vi "Autonomous Independent.vi"() -> ()   [LabVIEW 2016]
doc: "This VI is called when autonomous begins, and will automatically be terminated when autonomous ends. You can carry out timed or sensor driven robot movement independently without needing to return to the caller."
uses:
  AutoStates.ctl
  <vilib>/Platform/TimedLoop/XDataNode/timing_clust.ctl
  <vilib>/Platform/TimedLoop/XDataNode/nitl_modes.ctl
  <vilib>/Platform/TimedLoop/XDataNode/wakeup.ctl
  GearPositions.ctl
  Drive Commands.ctl
  Gear Command.ctl
  <vilib>/Rock Robotics/Network Tables/NT Read Number.vi
  <vilib>/Rock Robotics/Network Tables/NT Read Boolean.vi
  <vilib>/addons/control/pid/pid.llb/PID (DBL).vi
  <vilib>/platform/TimedLoop/XDataNode/XDataNode.xnode
  <vilib>/addons/control/pid/NI_PID_pid.lvlib
  <vilib>/Platform/TimedLoop/XDataNode/XDNodeRunTimeDep.lvlib
panel:
  in  "Orientation Limit":dbl=30.0
  out "Waveform Chart":cluster{i16, i16, i16}(graph)={1, 0, 0}
  in  "Drive Path Control":T1={"X"=[0.0, 26.0], "Y"=[0.0, 91.0], "Absolute Theta initial"=1.570796, "Absolute Theta final"=0.5016, "Amount of Time (s) 2"=3.0} {"Amount of Time (s) 2" format="%#_13g"}
  out "Arc Lenth Chart 2":cluster{dbl, "setpoint":dbl}(graph)={164.08658624999998, "setpoint"=169.64378866586094}
  out "Angle Chart (rad) 2":cluster{"Yaw Wind":dbl, "setpoint":dbl}(graph)={"Yaw Wind"=3.171890843977217, "setpoint"=3.2044361193738906}
  in  "Speed Range 2":cluster{"output high":dbl, "output low":dbl}={"output high"=1.0, "output low"=-1.0} {"output low" format="%.2f"; "output high" format="%.2f"}
  in  "PID Speed gains 2":T2={"proportional gain (Kc)"=0.1, "integral time (Ti, min)"=0.0, "derivative time (Td, min)"=0.0} {"derivative time (Td, min)" format="%.3f"; "integral time (Ti, min)" format="%.3f"; "proportional gain (Kc)" format="%.3f"}
  in  "Steer Range 2":cluster{"output high":dbl, "output low":dbl}={"output high"=1.0, "output low"=-1.0} {"output low" format="%.2f"; "output high" format="%.2f"}
  in  "Steer Gains":T2={"proportional gain (Kc)"=1.8, "integral time (Ti, min)"=0.0, "derivative time (Td, min)"=0.0} {"derivative time (Td, min)" format="%.3f"; "integral time (Ti, min)" format="%.3f"; "proportional gain (Kc)" format="%.3f"}
  in  "Eval Period (sec)":dbl(knob)=1.001252153636024 scale=0.0..1.5
  in  "PID Segments (1-500) 2":dbl=60.0
  out "Verify Graph 2":cluster{"X":dbl, "Y":dbl}[](graph)=[{"X"=0.0, "Y"=0.0}, {"X"=0.000288074563179022, "Y"=0.24281266883652286}, {"X"=0.0011475053216401378, "Y"=0.4902662165487718}, {"X"=0.0025713386426217373, "Y"=0.7423268407122737}, {"X"=0.004552620893362211, "Y"=0.9989607389025562}, {"X"=0.007084398441099949, "Y"=1.260134108695146}, {"X"=0.010159717653073339, "Y"=1.5258131476655705}, {"X"=0.013771624896520774, "Y"=1.795964053389357}, {"X"=0.017913166538680646, "Y"=2.0705530234420326}, {"X"=0.022577388946791337, "Y"=2.3495462553991238}, {"X"=0.027757338488091247, "Y"=2.632909946836159}, {"X"=0.03344606152981875, "Y"=2.9206102953286637}, {"X"=0.03963660443921224, "Y"=3.2126134984521664}, {"X"=0.046322013583510145, "Y"=3.5088857537821943}, {"X"=0.053495335329950794, "Y"=3.809393258894274}, {"X"=0.06114961604577262, "Y"=4.1141022113639325}, {"X"=0.06927790209821401, "Y"=4.422978808766698}, {"X"=0.07787323985451333, "Y"=4.735989248678097}, {"X"=0.08692867568190896, "Y"=5.053099728673654}, {"X"=0.09643725594763934, "Y"=5.374276446328901}, {"X"=0.10639202701894285, "Y"=5.699485599219363}, {"X"=0.1167860352630578, "Y"=6.028693384920565}, {"X"=0.1276123270472227, "Y"=6.36186600100804}, {"X"=0.13886394873867589, "Y"=6.698969645057309}, {"X"=0.15053394670465567, "Y"=7.0399705146439}, {"X"=0.1626153673124006, "Y"=7.384834807343345}, {"X"=0.17510125692914894, "Y"=7.733528720731165}, {"X"=0.18798466192213917, "Y"=8.086018452382891}, {"X"=0.20125862865860958, "Y"=8.442270199874049}, {"X"=0.21491620350579863, "Y"=8.802250160780169}, {"X"=0.2289504328309447, "Y"=9.16592453267677}, {"X"=0.24335436300128616, "Y"=9.533259513139388}, {"X"=0.2581210403840614, "Y"=9.904221299743547}, {"X"=0.27324351134650887, "Y"=10.278776090064776}, {"X"=0.2887148222558669, "Y"=10.656890081678597}, {"X"=0.3045280194793739, "Y"=11.038529472160542}, {"X"=0.32067614938426814, "Y"=11.423660459086133}, {"X"=0.33715225833778817, "Y"=11.812249240030901}, {"X"=0.3539493927071724, "Y"=12.204262012570375}, {"X"=0.37106059885965914, "Y"=12.599664974280081}, {"X"=0.38847892316248683, "Y"=12.998424322735545}, {"X"=0.4061974119828937, "Y"=13.400506255512294}, {"X"=0.4242091116881182, "Y"=13.805876970185853}, {"X"=0.44250706864539896, "Y"=14.214502664331752}, {"X"=0.4610843292219742, "Y"=14.626349535525518}, {"X"=0.4799339397850822, "Y"=15.04138378134268}, {"X"=0.49904894670196154, "Y"=15.45957159935876}, {"X"=0.5184223963398505, "Y"=15.88087918714929}, {"X"=0.5380473350659873, "Y"=16.305272742289795}, {"X"=0.5579168092476108, "Y"=16.732718462355802}, {"X"=0.5780238652519589, "Y"=17.16318254492284}, {"X"=0.5983615494462704, "Y"=17.596631187566434}, {"X"=0.6189229081977833, "Y"=18.03303058786211}, {"X"=0.6397009878737363, "Y"=18.4723469433854}, {"X"=0.6606888348413678, "Y"=18.91454645171183}, {"X"=0.6818794954679157, "Y"=19.35959531041692}, {"X"=0.7032660161206189, "Y"=19.807459717076206}, {"X"=0.7248414431667157, "Y"=20.258105869265208}, {"X"=0.7465988229734446, "Y"=20.711499964559465}, {"X"=0.7685312019080436, "Y"=21.16760820053449}, {"X"=0.7906316263377513, "Y"=21.62639677476582}, {"X"=0.812893142629806, "Y"=22.087831884828976}, {"X"=0.8353087971514465, "Y"=22.551879728299486}, {"X"=0.8578716362699106, "Y"=23.018506502752878}, {"X"=0.8805747063524371, "Y"=23.487678405764683}, {"X"=0.9034110537662644, "Y"=23.959361634910426}, {"X"=0.9263737248786306, "Y"=24.43352238776563}, {"X"=0.9494557660567741, "Y"=24.91012686190583}, {"X"=0.9726502236679336, "Y"=25.389141254906548}, {"X"=0.9959501440793475, "Y"=25.870531764343305}, {"X"=1.0193485736582537, "Y"=26.35426458779164}, {"X"=1.0428385587718907, "Y"=26.840305922827067}, {"X"=1.0664131457874975, "Y"=27.32862196702513}, {"X"=1.0900653810723118, "Y"=27.819178917961345}, {"X"=1.1137883109935727, "Y"=28.31194297321124}, {"X"=1.137574981918518, "Y"=28.806880330350346}, {"X"=1.161418440214386, "Y"=29.30395718695419}, {"X"=1.1853117322484152, "Y"=29.803139740598297}, {"X"=1.2092479043878446, "Y"=30.30439418885819}, {"X"=1.233220002999912, "Y"=30.807686729309403}, {"X"=1.2572210744518557, "Y"=31.312983559527456}, {"X"=1.2812441651109145, "Y"=31.820250877087886}, {"X"=1.3052823213443268, "Y"=32.329454879566214}, {"X"=1.3293285895193305, "Y"=32.84056176453797}, {"X"=1.3533760160031636, "Y"=33.35353772957866}, {"X"=1.3774176471630661, "Y"=33.86834897226385}, {"X"=1.4014465293662752, "Y"=34.38496169016904}, {"X"=1.4254557089800295, "Y"=34.90334208086977}, {"X"=1.4494382323715675, "Y"=35.42345634194157}, {"X"=1.4733871459081276, "Y"=35.94527067095994}, {"X"=1.497295495956948, "Y"=36.46875126550043}, {"X"=1.5211563288852672, "Y"=36.993864323138574}, {"X"=1.5449626910603236, "Y"=37.52057604144988}, {"X"=1.5687076288493556, "Y"=38.048852618009896}, {"X"=1.592384188619601, "Y"=38.578660250394115}, {"X"=1.6159854167382997, "Y"=39.1099651361781}, {"X"=1.6395043595726884, "Y"=39.64273347293735}, {"X"=1.6629340634900065, "Y"=40.176931458247424}, {"X"=1.6862675748574918, "Y"=40.712525289683825}, {"X"=1.7094979400423835, "Y"=41.249481164822086}, {"X"=1.7326182054119197, "Y"=41.78776528123773}, {"X"=1.7556214173333384, "Y"=42.3273438365063}, {"X"=1.778500622173878, "Y"=42.868183028203305}, {"X"=1.8012488663007775, "Y"=43.41024905390428}, {"X"=1.8238591960812744, "Y"=43.953508111184746}, {"X"=1.8463246578826074, "Y"=44.49792639762024}, {"X"=1.8686382980720155, "Y"=45.04347011078629}, {"X"=1.8907931630167365, "Y"=45.590105448258406}, {"X"=1.9127822990840087, "Y"=46.13779860761214}, {"X"=1.9345987526410706, "Y"=46.68651578642299}, {"X"=1.9562355700551612, "Y"=47.23622318226651}, {"X"=1.9776857976935183, "Y"=47.78688699271821}, {"X"=1.9989424819233803, "Y"=48.338473415353626}, {"X"=2.0199986691119856, "Y"=48.89094864774829}, {"X"=2.040847405626573, "Y"=49.44427888747771}, {"X"=2.06148173783438, "Y"=49.99843033211744}, {"X"=2.081894712102646, "Y"=50.55336917924298}, {"X"=2.102079374798609, "Y"=51.10906162642988}, {"X"=2.1220287722895073, "Y"=51.665473871253646}, {"X"=2.141735950942579, "Y"=52.22257211128982}, {"X"=2.1611939571250627, "Y"=52.78032254411392}, {"X"=2.1803958372041974, "Y"=53.33869136730149}, {"X"=2.1993346375472207, "Y"=53.897644778428024}, {"X"=2.218003404521371, "Y"=54.457148975069096}, {"X"=2.2363951844938876, "Y"=55.0171701548002}, {"X"=2.2545030238320076, "Y"=55.577674515196854}, {"X"=2.2723199689029703, "Y"=56.13862825383462}, {"X"=2.289839066074014, "Y"=56.699997568289}, {"X"=2.3070533617123767, "Y"=57.26174865613553}, {"X"=2.3239559021852974, "Y"=57.82384771494973}, {"X"=2.340539733860014, "Y"=58.38626094230713}, {"X"=2.3567979031037645, "Y"=58.94895453578327}, {"X"=2.3727234562837882, "Y"=59.51189469295367}, {"X"=2.3883094397673226, "Y"=60.07504761139384}, {"X"=2.4035488999216073, "Y"=60.63837948867933}, {"X"=2.41843488311388, "Y"=61.201856522385654}, {"X"=2.4329604357113785, "Y"=61.76544491008834}, {"X"=2.447118604081342, "Y"=62.32911084936293}, {"X"=2.460902434591008, "Y"=62.892820537784935}, {"X"=2.4743049736076164, "Y"=63.456540172929884}, {"X"=2.487319267498404, "Y"=64.0202359523733}, {"X"=2.49993836263061, "Y"=64.58387407369071}, {"X"=2.512155305371473, "Y"=65.14742073445767}, {"X"=2.523963142088231, "Y"=65.71084213224968}, {"X"=2.5353549191481224, "Y"=66.27410446464226}, {"X"=2.546323682918386, "Y"=66.83717392921096}, {"X"=2.55686247976626, "Y"=67.40001672353131}, {"X"=2.566964356058982, "Y"=67.9625990451788}, {"X"=2.576622358163791, "Y"=68.524887091729}, {"X"=2.5858295324479257, "Y"=69.0868470607574}, {"X"=2.5945789252786247, "Y"=69.64844514983957}, {"X"=2.6028635830231246, "Y"=70.209647556551}, {"X"=2.610676552048666, "Y"=70.77042047846723}, {"X"=2.618010878722486, "Y"=71.3307301131638}, {"X"=2.6248596094118235, "Y"=71.8905426582162}, {"X"=2.6312157904839166, "Y"=72.44982431119999}, {"X"=2.6370724683060045, "Y"=73.0085412696907}, {"X"=2.642422689245324, "Y"=73.56665973126384}, {"X"=2.6472594996691154, "Y"=74.12414589349494}, {"X"=2.651575945944615, "Y"=74.68096595395953}, {"X"=2.655365074439064, "Y"=75.23708611023312}, {"X"=2.658619931519697, "Y"=75.79247255989128}, {"X"=2.661333563553756, "Y"=76.3470915005095}, {"X"=2.663499016908478, "Y"=76.90090912966333}, {"X"=2.6651093379510997, "Y"=77.45389164492828}, {"X"=2.6661575730488627, "Y"=78.00600524387988}, {"X"=2.6666367685690027, "Y"=78.55721612409367}, {"X"=2.6665399708787594, "Y"=79.10749048314513}, {"X"=2.665860226345371, "Y"=79.65679451860986}, {"X"=2.664590581336076, "Y"=80.20509442806333}, {"X"=2.6627240822181117, "Y"=80.75235640908112}, {"X"=2.6602537753587185, "Y"=81.2985466592387}, {"X"=2.657172707125133, "Y"=81.84363137611163}, {"X"=2.653473923884595, "Y"=82.38757675727544}, {"X"=2.649150472004342, "Y"=82.93034900030563}, {"X"=2.644195397851612, "Y"=83.47191430277776}, {"X"=2.6386017477936443, "Y"=84.01223886226732}, {"X"=2.6323625681976766, "Y"=84.55128887634989}, {"X"=2.6254709054309484, "Y"=85.08903054260095}, {"X"=2.617919805860696, "Y"=85.62543005859604}, {"X"=2.60970231585416, "Y"=86.1604536219107}, {"X"=2.6008114817785777, "Y"=86.69406743012043}, {"X"=2.591240350001188, "Y"=87.22623768080079}, {"X"=2.580981966889228, "Y"=87.75693057152729}, {"X"=2.570029378809939, "Y"=88.28611229987547}, {"X"=2.5583756321305553, "Y"=88.81374906342081}, {"X"=2.546013773218319, "Y"=89.33980705973892}, {"X"=2.5329368484404657, "Y"=89.86425248640526}, {"X"=2.5191379041642357, "Y"=90.38705154099536}, {"X"=2.5046099867568676, "Y"=90.90817042108478}, {"X"=2.489346142585597, "Y"=91.42757532424903}, {"X"=2.4733394180176655, "Y"=91.94523244806365}, {"X"=2.4565828594203096, "Y"=92.46110799010413}, {"X"=2.4390695131607694, "Y"=92.97516814794604}, {"X"=2.4207924256062805, "Y"=93.4873791191649}, {"X"=2.401744643124084, "Y"=93.99770710133622}, {"X"=2.3819192120814163, "Y"=94.50611829203552}, {"X"=2.3613091788455183, "Y"=95.01257888883835}, {"X"=2.3399075897836252, "Y"=95.51705508932024}, {"X"=2.3177074912629783, "Y"=96.0195130910567}, {"X"=2.2947019296508144, "Y"=96.51991909162327}, {"X"=2.2708839513143713, "Y"=97.01823928859547}, {"X"=2.246246602620889, "Y"=97.51443987954882}, {"X"=2.220782929937605, "Y"=98.00848706205885}, {"X"=2.194485979631758, "Y"=98.5003470337011}, {"X"=2.1673487980705857, "Y"=98.98998599205109}, {"X"=2.139364431621328, "Y"=99.47737013468435}, {"X"=2.110525926651221, "Y"=99.9624656591764}, {"X"=2.080826329527506, "Y"=100.44523876310278}, {"X"=2.0502586866174184, "Y"=100.92565564403898}, {"X"=2.018816044288199, "Y"=101.40368249956057}, {"X"=1.9864914489070844, "Y"=101.87928552724307}, {"X"=1.9532779468413146, "Y"=102.352430924662}, {"X"=1.9191685844581259, "Y"=102.82308488939287}, {"X"=1.8841564081247597, "Y"=103.29121361901124}, {"X"=1.8482344642084523, "Y"=103.75678331109262}, {"X"=1.811395799076441, "Y"=104.21976016321254}, {"X"=1.7736334590959675, "Y"=104.68011037294652}, {"X"=1.7349404906342674, "Y"=105.13780013787007}, {"X"=1.6953099400585805, "Y"=105.59279565555877}, {"X"=1.6547348537361435, "Y"=106.04506312358811}, {"X"=1.6132082780341972, "Y"=106.49456873953362}, {"X"=1.5707232593199776, "Y"=106.94127870097084}, {"X"=1.5272728439607242, "Y"=107.38515920547528}, {"X"=1.4828500783236782, "Y"=107.82617645062247}, {"X"=1.4374480087760724, "Y"=108.26429663398795}, {"X"=1.3910596816851482, "Y"=108.69948595314725}, {"X"=1.3436781434181464, "Y"=109.13171060567588}, {"X"=1.2952964403423002, "Y"=109.56093678914935}, {"X"=1.2459076188248506, "Y"=109.98713070114324}, {"X"=1.1955047252330357, "Y"=110.41025853923304}, {"X"=1.1440808059340977, "Y"=110.83028650099428}, {"X"=1.091628907295268, "Y"=111.24718078400251}, {"X"=1.0381420756837887, "Y"=111.66090758583321}, {"X"=0.9836133574668977, "Y"=112.07143310406197}, {"X"=0.9280357990118371, "Y"=112.47872353626427}, {"X"=0.8714024466858384, "Y"=112.88274508001565}, {"X"=0.8137063468561436, "Y"=113.28346393289164}, {"X"=0.7549405458899908, "Y"=113.68084629246776}, {"X"=0.6950980901546219, "Y"=114.07485835631954}, {"X"=0.6341720260172685, "Y"=114.46546632202252}, {"X"=0.5721553998451724, "Y"=114.85263638715222}, {"X"=0.5090412580055753, "Y"=115.23633474928415}, {"X"=0.4448226468657089, "Y"=115.61652760599387}, {"X"=0.37949261279281826, "Y"=115.99318115485687}, {"X"=0.31304420215413525, "Y"=116.3662615934487}, {"X"=0.24547046131690142, "Y"=116.73573511934488}, {"X"=0.17676443664835523, "Y"=117.10156793012095}, {"X"=0.10691917451573854, "Y"=117.46372622335241}, {"X"=0.03592772128628276, "Y"=117.82217619661483}, {"X"=-0.036216651323535125, "Y"=118.17688514203918}, {"X"=-0.10951548856480563, "Y"=118.52784552653254}, {"X"=-0.18396515265619237, "Y"=118.87507499177802}, {"X"=-0.25956178046712086, "Y"=119.21859227401423}, {"X"=-0.3363015088670166, "Y"=119.55841610947977}, {"X"=-0.414180474725305, "Y"=119.89456523441324}, {"X"=-0.4931948149114117, "Y"=120.22705838505323}, {"X"=-0.5733406662947621, "Y"=120.55591429763835}, {"X"=-0.6546141657447817, "Y"=120.8811517084072}, {"X"=-0.737011450130896, "Y"=121.20278935359838}, {"X"=-0.8205286563225305, "Y"=121.52084596945049}, {"X"=-0.9051619211891107, "Y"=121.83534029220215}, {"X"=-0.990907381600062, "Y"=122.14629105809192}, {"X"=-1.07776117442481, "Y"=122.45371700335843}, {"X"=-1.16571943653278, "Y"=122.75763686424028}, {"X"=-1.254778304793398, "Y"=123.05806937697606}, {"X"=-1.3449339160760891, "Y"=123.35503327780438}, {"X"=-1.4361824072502785, "Y"=123.64854730296383}, {"X"=-1.5285199151853923, "Y"=123.93863018869303}, {"X"=-1.6219425767508557, "Y"=124.22530067123054}, {"X"=-1.7164465288160942, "Y"=124.50857748681501}, {"X"=-1.8120279082505333, "Y"=124.78847937168501}, {"X"=-1.9086828519235983, "Y"=125.06502506207916}, {"X"=-2.0064074967047154, "Y"=125.33823329423605}, {"X"=-2.105197979463309, "Y"=125.60812280439427}, {"X"=-2.2050504370688055, "Y"=125.87471232879243}, {"X"=-2.30596100639063, "Y"=126.13802060366913}, {"X"=-2.407925824298208, "Y"=126.39806636526299}, {"X"=-2.5109410276609654, "Y"=126.65486834981257}, {"X"=-2.615002753348327, "Y"=126.90844529355651}, {"X"=-2.720107138229719, "Y"=127.15881593273339}, {"X"=-2.8262503191745663, "Y"=127.40599900358183}, {"X"=-2.933428433052288, "Y"=127.65001324234038}, {"X"=-3.0416376167323227, "Y"=127.8908773852477}, {"X"=-3.1508740070840897, "Y"=128.12861016854237}, {"X"=-3.261133740977014, "Y"=128.36323032846298}, {"X"=-3.3724129552805215, "Y"=128.59475660124815}, {"X"=-3.4847077868640373, "Y"=128.82320772313645}, {"X"=-3.5980143725969866, "Y"=129.04860243036651}, {"X"=-3.712328849348796, "Y"=129.27095945917694}, {"X"=-3.8276473539888904, "Y"=129.4902975458063}, {"X"=-3.9439660233866953, "Y"=129.70663542649322}, {"X"=-4.061280994411636, "Y"=129.9199918374763}, {"X"=-4.1795884039331375, "Y"=130.1303855149941}, {"X"=-4.2988843888206265, "Y"=130.33783519528527}, {"X"=-4.419165085943527, "Y"=130.5423596145884}, {"X"=-4.540426632171267, "Y"=130.7439775091421}, {"X"=-4.66266516437327, "Y"=130.94270761518493}, {"X"=-4.785876819418961, "Y"=131.13856866895551}, {"X"=-4.910057734177768, "Y"=131.33157940669247}, {"X"=-5.035204045519113, "Y"=131.52175856463438}, {"X"=-5.161311890312425, "Y"=131.70912487901987}, {"X"=-5.288377405427127, "Y"=131.89369708608749}, {"X"=-5.4163967277326455, "Y"=132.07549392207588}, {"X"=-5.545365994098406, "Y"=132.25453412322364}, {"X"=-5.675281341393834, "Y"=132.43083642576934}, {"X"=-5.806138906488355, "Y"=132.60441956595162}, {"X"=-5.937934826251394, "Y"=132.77530228000904}, {"X"=-6.070665237552376, "Y"=132.94350330418024}, {"X"=-6.204326277260728, "Y"=133.10904137470382}, {"X"=-6.338914082245876, "Y"=133.27193522781835}, {"X"=-6.474424789377243, "Y"=133.43220359976243}, {"X"=-6.610854535524256, "Y"=133.5898652267747}, {"X"=-6.74819945755634, "Y"=133.7449388450937}, {"X"=-6.886455692342921, "Y"=133.8974431909581}, {"X"=-7.025619376753425, "Y"=134.04739700060648}, {"X"=-7.165686647657276, "Y"=134.1948190102774}, {"X"=-7.3066536419239005, "Y"=134.3397279562095}, {"X"=-7.448516496422724, "Y"=134.48214257464136}, {"X"=-7.591271348023172, "Y"=134.6220816018116}, {"X"=-7.734914333594669, "Y"=134.7595637739588}, {"X"=-7.879441590006641, "Y"=134.89460782732158}, {"X"=-8.024849254128513, "Y"=135.02723249813855}, {"X"=-8.171133462829713, "Y"=135.15745652264826}, {"X"=-8.318290352979664, "Y"=135.28529863708937}, {"X"=-8.466316061447793, "Y"=135.41077757770046}, {"X"=-8.615206725103523, "Y"=135.53391208072009}, {"X"=-8.764958480816283, "Y"=135.65472088238693}, {"X"=-8.915567465455496, "Y"=135.77322271893954}, {"X"=-9.067029815890589, "Y"=135.8894363266165}, {"X"=-9.219341668990985, "Y"=136.00338044165647}, {"X"=-9.372499161626111, "Y"=136.115073800298}, {"X"=-9.526498430665395, "Y"=136.22453513877971}, {"X"=-9.68133561297825, "Y"=136.3317831933402}, {"X"=-9.83700684543412, "Y"=136.43683670021807}, {"X"=-9.993508264902422, "Y"=136.5397143956519}, {"X"=-10.150836008252583, "Y"=136.64043501588037}, {"X"=-10.308986212354027, "Y"=136.73901729714197}, {"X"=-10.467955014076177, "Y"=136.83547997567538}, {"X"=-10.627738550288464, "Y"=136.92984178771917}, {"X"=-10.788332957860309, "Y"=137.02212146951194}, {"X"=-10.94973437366114, "Y"=137.1123377572923}, {"X"=-11.111938934560381, "Y"=137.20050938729884}, {"X"=-11.274942777427457, "Y"=137.28665509577016}, {"X"=-11.438742039131796, "Y"=137.37079361894487}, {"X"=-11.603332856542822, "Y"=137.45294369306157}, {"X"=-11.76871136652996, "Y"=137.53312405435886}, {"X"=-11.934873705962637, "Y"=137.61135343907534}, {"X"=-12.101816011710278, "Y"=137.68765058344962}, {"X"=-12.269534420642309, "Y"=137.7620342237203}, {"X"=-12.438025069628152, "Y"=137.83452309612593}, {"X"=-12.607284095537233, "Y"=137.90513593690517}, {"X"=-12.777307635238984, "Y"=137.9738914822966}, {"X"=-12.948091825602823, "Y"=138.04080846853884}, {"X"=-13.11963280349818, "Y"=138.10590563187046}, {"X"=-13.291926705794477, "Y"=138.16920170853007}, {"X"=-13.464969669361142, "Y"=138.2307154347563}, {"X"=-13.638757831067604, "Y"=138.2904655467877}, {"X"=-13.81328732778328, "Y"=138.3484707808629}, {"X"=-13.988554296377602, "Y"=138.4047498732205}, {"X"=-14.164554873719993, "Y"=138.45932156009908}, {"X"=-14.341285196679879, "Y"=138.5122045777373}, {"X"=-14.518741402126686, "Y"=138.5634176623737}, {"X"=-14.696919626929835, "Y"=138.61297955024688}, {"X"=-14.87581600795876, "Y"=138.66090897759548}, {"X"=-15.05542668208288, "Y"=138.70722468065807}, {"X"=-15.235747786171622, "Y"=138.75194539567326}, {"X"=-15.416775457094413, "Y"=138.79508985887966}, {"X"=-15.598505831720678, "Y"=138.83667680651587}, {"X"=-15.78093504691984, "Y"=138.87672497482046}, {"X"=-15.964059239561328, "Y"=138.9152531000321}, {"X"=-16.147874546514565, "Y"=138.95227991838928}, {"X"=-16.332377104648977, "Y"=138.9878241661307}, {"X"=-16.517563050833992, "Y"=139.02190457949493}, {"X"=-16.70342852193903, "Y"=139.05453989472056}, {"X"=-16.889969654833525, "Y"=139.08574884804622}, {"X"=-17.077182586386893, "Y"=139.11555017571047}, {"X"=-17.265063453468567, "Y"=139.1439626139519}, {"X"=-17.453608392947967, "Y"=139.17100489900918}, {"X"=-17.64281354169452, "Y"=139.19669576712087}, {"X"=-17.832675036577655, "Y"=139.22105395452556}, {"X"=-18.02318901446679, "Y"=139.24409819746185}, {"X"=-18.214351612231358, "Y"=139.26584723216837}, {"X"=-18.406158966740783, "Y"=139.2863197948837}, {"X"=-18.59860721486448, "Y"=139.30553462184642}, {"X"=-18.79169249347189, "Y"=139.32351044929518}, {"X"=-18.985410939432434, "Y"=139.34026601346855}, {"X"=-19.179758689615536, "Y"=139.35582005060513}, {"X"=-19.37473188089062, "Y"=139.37019129694355}, {"X"=-19.570326650127114, "Y"=139.38339848872235}, {"X"=-19.766539134194442, "Y"=139.3954603621802}, {"X"=-19.96336546996203, "Y"=139.40639565355565}, {"X"=-20.160801794299303, "Y"=139.41622309908732}, {"X"=-20.35884424407569, "Y"=139.4249614350138}, {"X"=-20.557488956160604, "Y"=139.43262939757372}, {"X"=-20.756732067423485, "Y"=139.43924572300563}, {"X"=-20.956569714733757, "Y"=139.4448291475482}, {"X"=-21.15699803496084, "Y"=139.44939840743996}, {"X"=-21.35801316497416, "Y"=139.45297223891956}, {"X"=-21.55961124164314, "Y"=139.4555693782256}, {"X"=-21.76178840183722, "Y"=139.45720856159664}, {"X"=-21.964540782425804, "Y"=139.4579085252713}, {"X"=-22.167864520278332, "Y"=139.4576880054882}, {"X"=-22.37175575226422, "Y"=139.45656573848592}, {"X"=-22.576210615252908, "Y"=139.45456046050307}, {"X"=-22.781225246113806, "Y"=139.45169090777824}, {"X"=-22.986795781716346, "Y"=139.44797581655004}, {"X"=-23.19291835892996, "Y"=139.44343392305709}, {"X"=-23.399589114624064, "Y"=139.43808396353793}, {"X"=-23.606804185668086, "Y"=139.43194467423123}, {"X"=-23.814559708931448, "Y"=139.42503479137557}, {"X"=-24.022851821283584, "Y"=139.41737305120952}, {"X"=-24.231676659593916, "Y"=139.4089781899717}, {"X"=-24.44103036073187, "Y"=139.3998689439007}, {"X"=-24.650909061566864, "Y"=139.39006404923518}, {"X"=-24.861308898968336, "Y"=139.37958224221367}, {"X"=-25.0722260098057, "Y"=139.36844225907478}, {"X"=-25.28365653094839, "Y"=139.35666283605715}, {"X"=-25.495596599265824, "Y"=139.34426270939935}, {"X"=-25.708042351627437, "Y"=139.33126061533997}, {"X"=-25.92098992490265, "Y"=139.31767529011762}, {"X"=-26.13443545596088, "Y"=139.30352546997094}, {"X"=-26.348375081671563, "Y"=139.28882989113848}, {"X"=-26.56280493890412, "Y"=139.27360728985886}, {"X"=-26.777721164527982, "Y"=139.2578764023707}, {"X"=-26.99311989541257, "Y"=139.24165596491255}, {"X"=-27.208997268427304, "Y"=139.22496471372307}, {"X"=-27.425349420441623, "Y"=139.2078213850408}, {"X"=-27.64217248832494, "Y"=139.1902447151044}, {"X"=-27.85946260894669, "Y"=139.17225344015242}, {"X"=-28.07721591917629, "Y"=139.1538662964235}, {"X"=-28.295428555883166, "Y"=139.13510202015624}, {"X"=-28.514096655936754, "Y"=139.1159793475892}, {"X"=-28.73321635620647, "Y"=139.096517014961}, {"X"=-28.95278379356174, "Y"=139.07673375851027}, {"X"=-29.172795104871994, "Y"=139.05664831447558}, {"X"=-29.393246427006645, "Y"=139.03627941909554}, {"X"=-29.614133896835135, "Y"=139.01564580860872}, {"X"=-29.835453651226885, "Y"=138.9947662192538}, {"X"=-30.05720182705132, "Y"=138.9736593872693}, {"X"=-30.279374561177864, "Y"=138.95234404889385}, {"X"=-30.501967990475933, "Y"=138.93083894036604}, {"X"=-30.72497825181497, "Y"=138.90916279792452}, {"X"=-30.94840148206439, "Y"=138.88733435780782}, {"X"=-31.17223381809363, "Y"=138.86537235625457}, {"X"=-31.3964713967721, "Y"=138.8432955295034}, {"X"=-31.62111035496923, "Y"=138.82112261379285}, {"X"=-31.846146829554442, "Y"=138.79887234536162}, {"X"=-32.07157695739718, "Y"=138.7765634604482}, {"X"=-32.29739687536684, "Y"=138.7542146952912}, {"X"=-32.52360272033288, "Y"=138.73184478612933}, {"X"=-32.7501906291647, "Y"=138.70947246920107}, {"X"=-32.977156738731736, "Y"=138.6871164807451}, {"X"=-33.20449718590342, "Y"=138.66479555699996}, {"X"=-33.43220810754916, "Y"=138.64252843420428}, {"X"=-33.66028564053839, "Y"=138.6203338485967}, {"X"=-33.888725921740544, "Y"=138.59823053641574}, {"X"=-34.11752508802504, "Y"=138.57623723390006}, {"X"=-34.3466792762613, "Y"=138.55437267728823}, {"X"=-34.576184623318746, "Y"=138.53265560281886}, {"X"=-34.806037266066824, "Y"=138.51110474673058}, {"X"=-35.03623334137494, "Y"=138.48973884526194}, {"X"=-35.26676898611253, "Y"=138.46857663465158}, {"X"=-35.49764033714901, "Y"=138.44763685113807}, {"X"=-35.72884353135381, "Y"=138.42693823096005}, {"X"=-35.96037470559636, "Y"=138.4064995103561}, {"X"=-36.19222999674608, "Y"=138.38633942556478}, {"X"=-36.4244055416724, "Y"=138.36647671282475}, {"X"=-36.65689747724474, "Y"=138.3469301083746}, {"X"=-36.88970194033253, "Y"=138.32771834845292}, {"X"=-37.12281506780519, "Y"=138.3088601692983}, {"X"=-37.35623299653215, "Y"=138.29037430714936}, {"X"=-37.58995186338284, "Y"=138.27227949824467}, {"X"=-37.82396780522667, "Y"=138.25459447882287}, {"X"=-38.05827695893308, "Y"=138.23733798512254}, {"X"=-38.292875461371494, "Y"=138.22052875338227}, {"X"=-38.527759449411334, "Y"=138.2041855198407}, {"X"=-38.76292505992202, "Y"=138.18832702073638}, {"X"=-38.998368429773, "Y"=138.17297199230796}, {"X"=-39.23408569583366, "Y"=138.15813917079402}, {"X"=-39.470072994973464, "Y"=138.14384729243312}, {"X"=-39.70632646406182, "Y"=138.13011509346393}, {"X"=-39.94284223996815, "Y"=138.11696131012502}, {"X"=-40.17961645956189, "Y"=138.10440467865496}, {"X"=-40.41664525971246, "Y"=138.09246393529241}, {"X"=-40.65392477728929, "Y"=138.08115781627595}, {"X"=-40.891451149161796, "Y"=138.07050505784412}, {"X"=-41.129220512199396, "Y"=138.0605243962356}, {"X"=-41.36722900327154, "Y"=138.05123456768897}, {"X"=-41.60547275924765, "Y"=138.04265430844282}, {"X"=-41.84394791699713, "Y"=138.03480235473575}, {"X"=-42.08265061338943, "Y"=138.02769744280636}, {"X"=-42.32157698529396, "Y"=138.02135830889327}, {"X"=-42.56072316958015, "Y"=138.01580368923504}, {"X"=-42.800085303117434, "Y"=138.01105232007032}, {"X"=-43.039659522775224, "Y"=138.0071229376377}, {"X"=-43.27944196542294, "Y"=138.0040342781757}, {"X"=-43.51942876793002, "Y"=138.00180507792305}, {"X"=-43.7596160671659, "Y"=138.00045407311828}, {"X"=-44.0, "Y"=138.0}]
  # "Be sure to right-click and choose Data Operations>>Make Current Value default if you want to save the array values with the VI"
  # "(73)"
  # "(64)"
  # "(48)"
  # "(76)"
  # "(64)"
  # "0.8"
  # "0.5 Right"
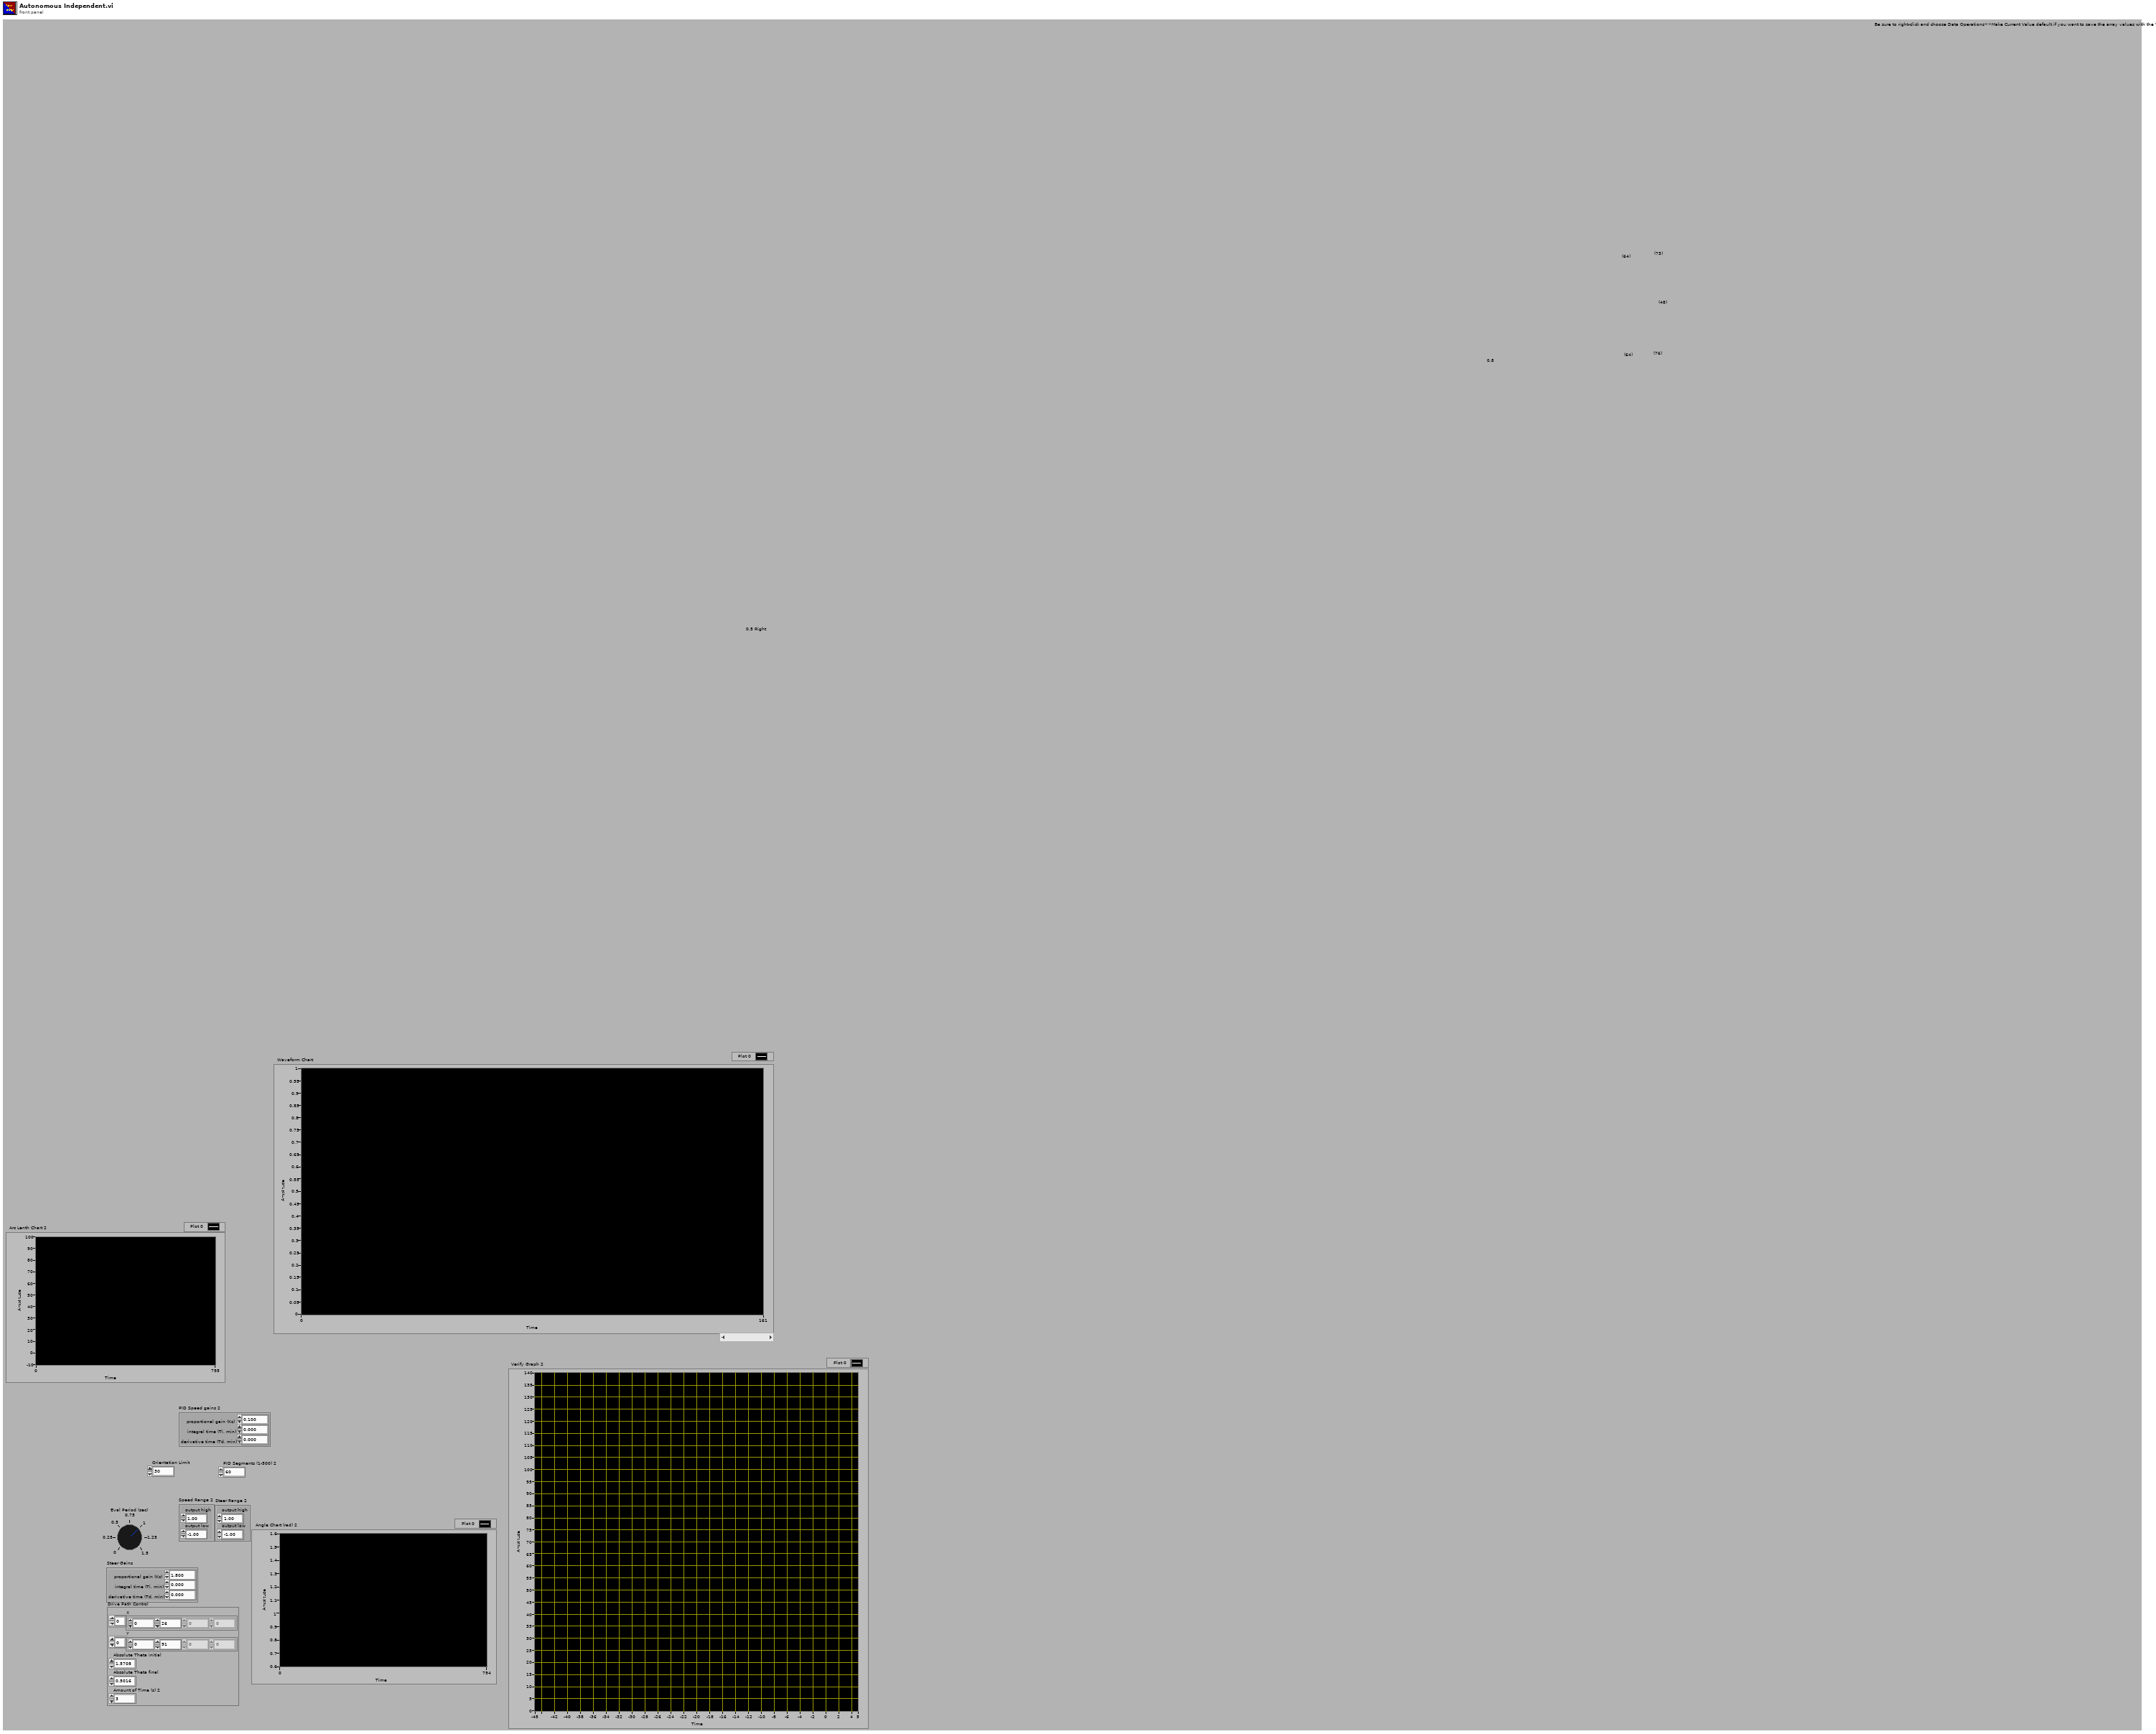
[diagram p1: front panel]
types:
  T1 = cluster{"X":dbl[], "Y":dbl[], "Absolute Theta initial":dbl, "Absolute Theta final":dbl, "Amount of Time (s) 2":dbl}
  T2 = cluster{"proportional gain (Kc)":dbl, "integral time (Ti, min)":dbl, "derivative time (Td, min)":dbl}
  T3 = typedef "GearPositions.ctl" = enum16{"Left", "Center", "Right"}
  T4 = cluster{"Body IMU":dbl, "Right Encoder Init":dbl, "Left Encoder Init":dbl, "Gear":bool, "Peg":T3, "Initial Time":u32, "Shoot ASAP!":bool}
  T5 = cluster{"X":dbl[], "Y":dbl[], "Absolute Theta initial":dbl, "Absolute Theta final":dbl}
  T6 = typedef "AutoStates.ctl" = enum16{"Calculate Path", "Drive Path", "Gear Cam Placement", "Hopper Shoot", "Leave Peg", "Crash Adjustment", "Early Left Shot"}
  T7 = typedef "XDNodeRunTimeDep.lvlib/timing_clust.ctl" = cluster{"Expected End [f-1]":u64, "Actual End [f-1]":u64, "Finished Late? [f-1]":bool, "Expected End [i-1]":u64, "Actual End [i-1]":u64, "Finished Late? [i-1]":bool, "Expected Start [i]":u64, "Actual Start [i]":u64, "Expected Start [f]":u64, "Actual Start [f]":u64, "Source Name":string, "Structure Name":string, "Period":i64, "Deadline":i64, "Offset":i64, "Start":i64, "Priority":i32, "Timeout":i32, "Mode":T8, "Wakeup Reason":T9, "Error":errorcluster, "Source Type":string, "Secondary Source Type":string, "Global End Time":u64, "Global Start Time":u64, "Frame Duration":u64, "Iteration Duration":u64, "Assigned CPU":i32, "I/O Scan Engine Mode":u32}
  T8 = typedef "XDNodeRunTimeDep.lvlib/nitl_modes.ctl" = enum32{"No Change", "Process missed periods, maintain original phase", "Discard missed periods, maintain original phase", "Process missed periods, ignore original phase", "Discard missed periods, ignore original phase"}
  T9 = typedef "XDNodeRunTimeDep.lvlib/wakeup.ctl" = enum32{"Normal", "Aborted", "Asynchronous wakeup", "Timing source error", "Timed loop error", "Timeout"}
  T10 = typedef "Drive Commands.ctl" = enum16{"Manual", "Get Gear", "Score Gear", "Align Rope", "Turn To Angle", "Start Gear Score", "Place Gear", "Tank Drive", "Drive Distance"}
  T11 = typedef "Gear Command.ctl" = enum16{"Home", "Floor Intake", "Catch", "Score"}
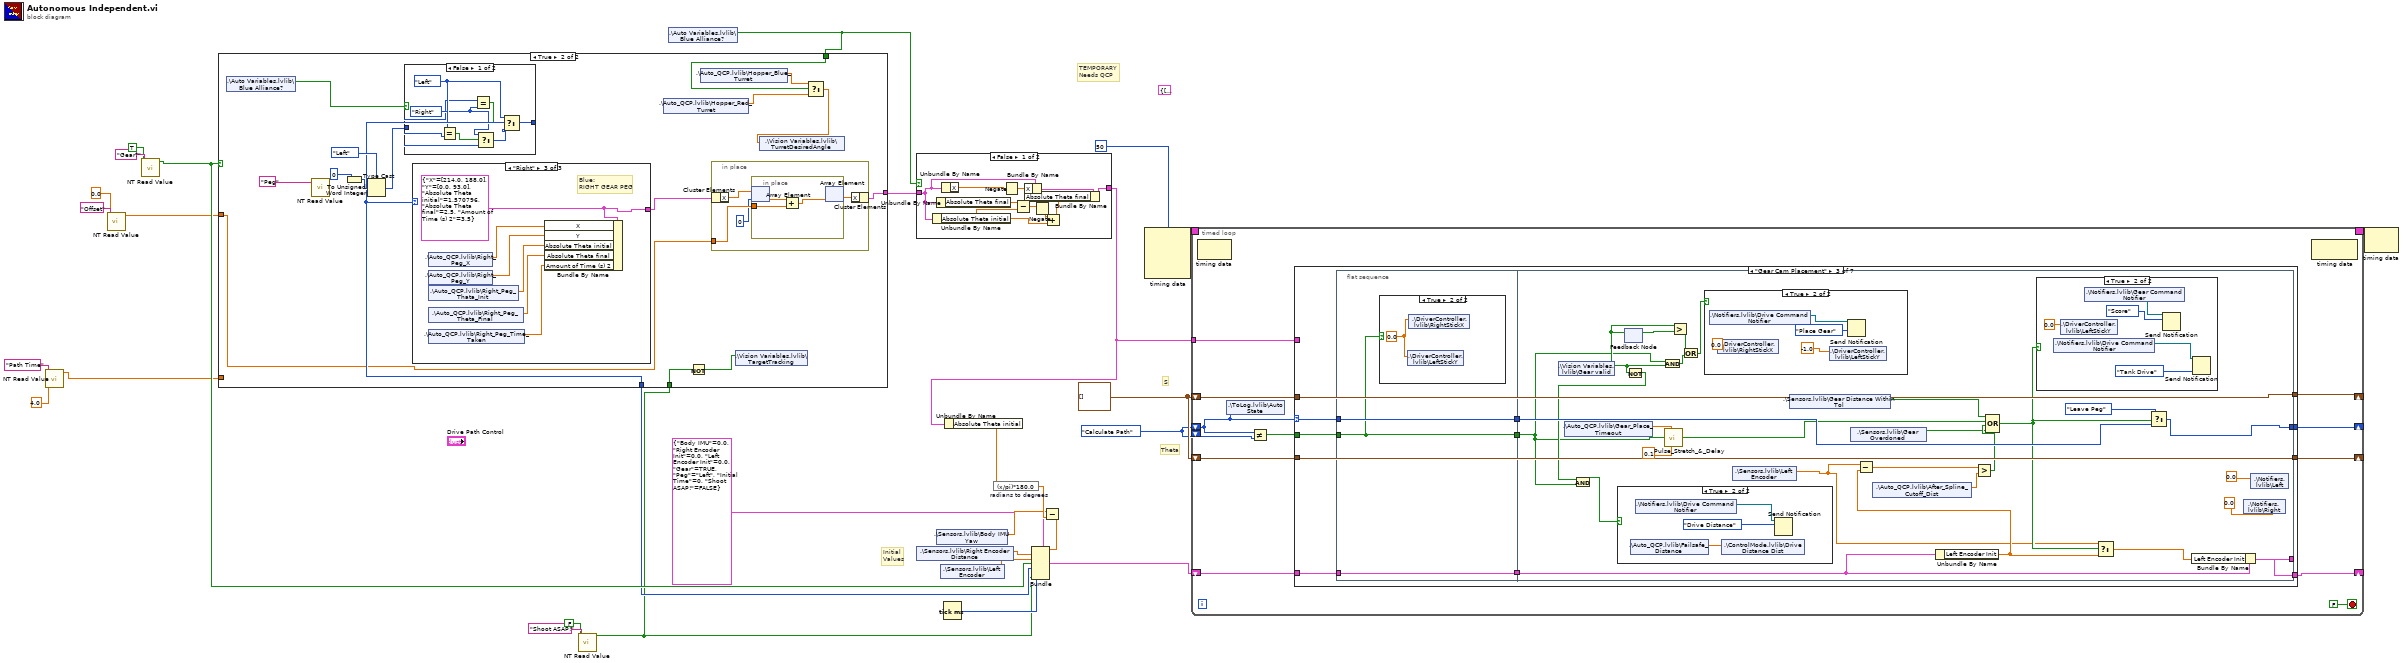
[diagram p0: block diagram]
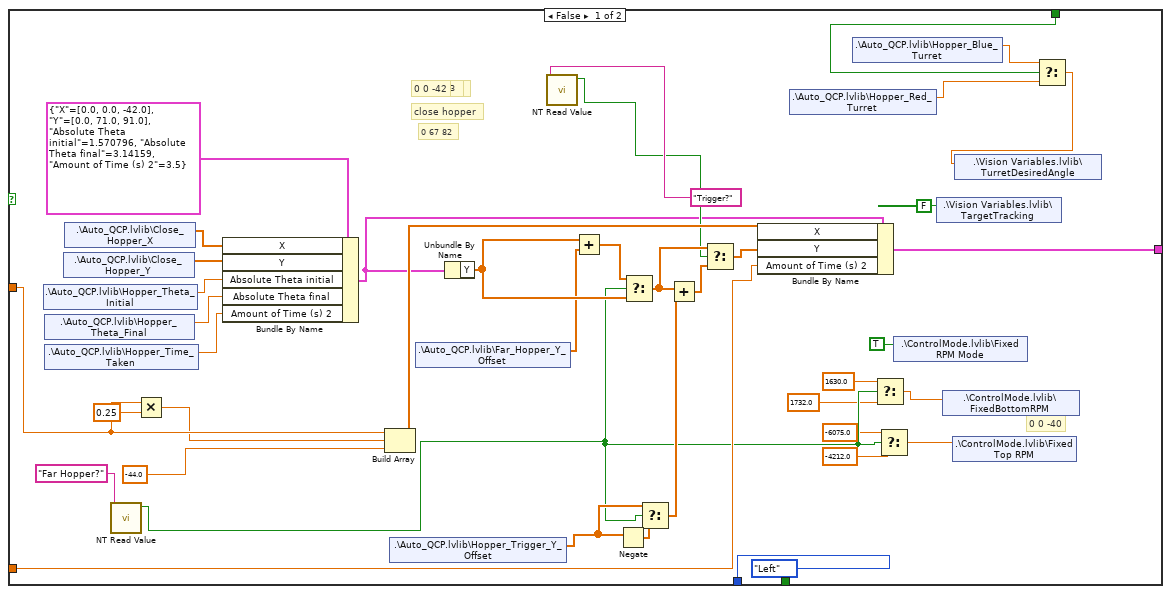
[diagram p2: hidden frame]
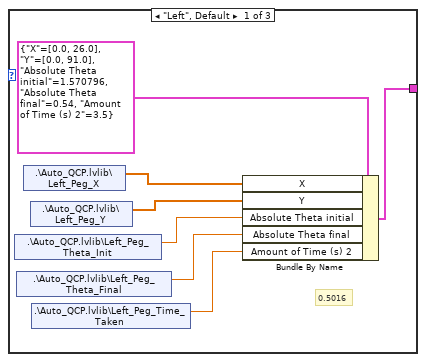
[diagram p4: hidden frame]
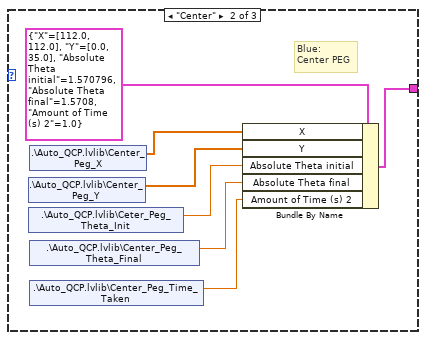
[diagram p5: hidden frame]
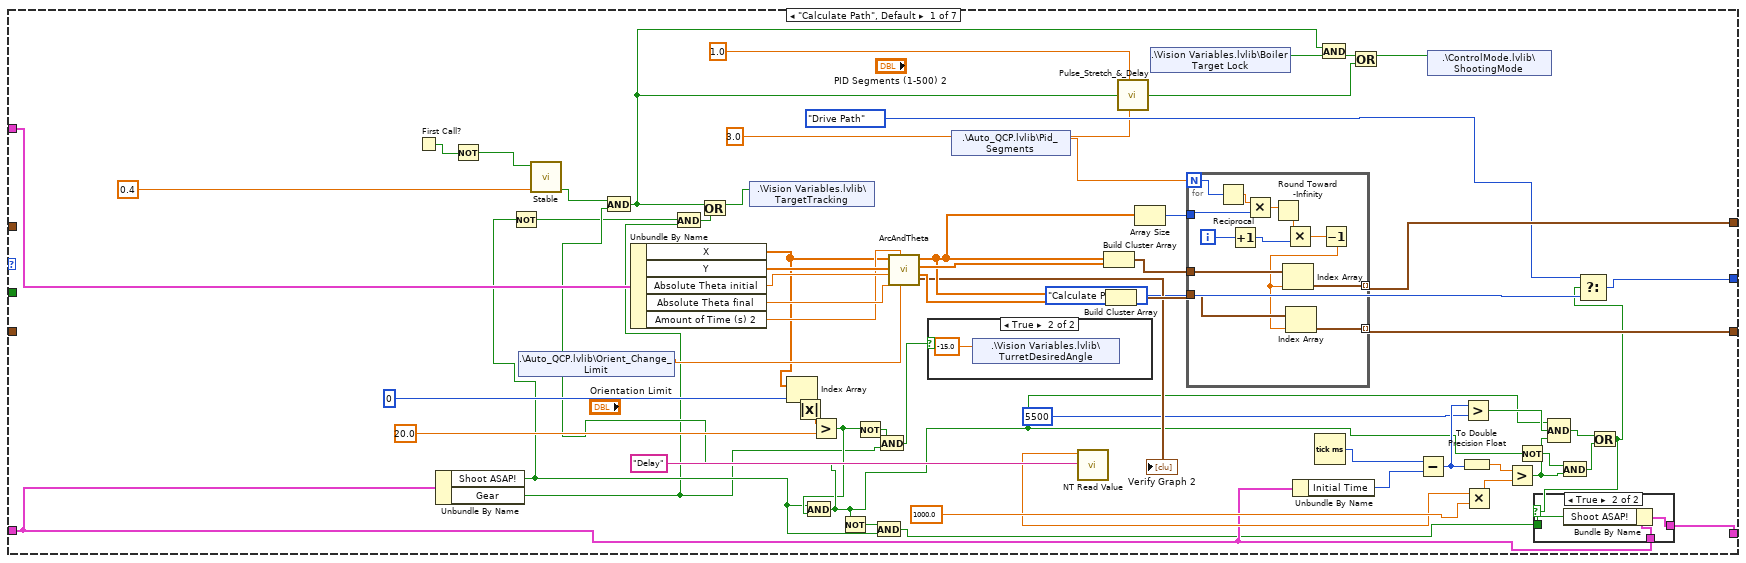
[diagram p7: hidden frame]
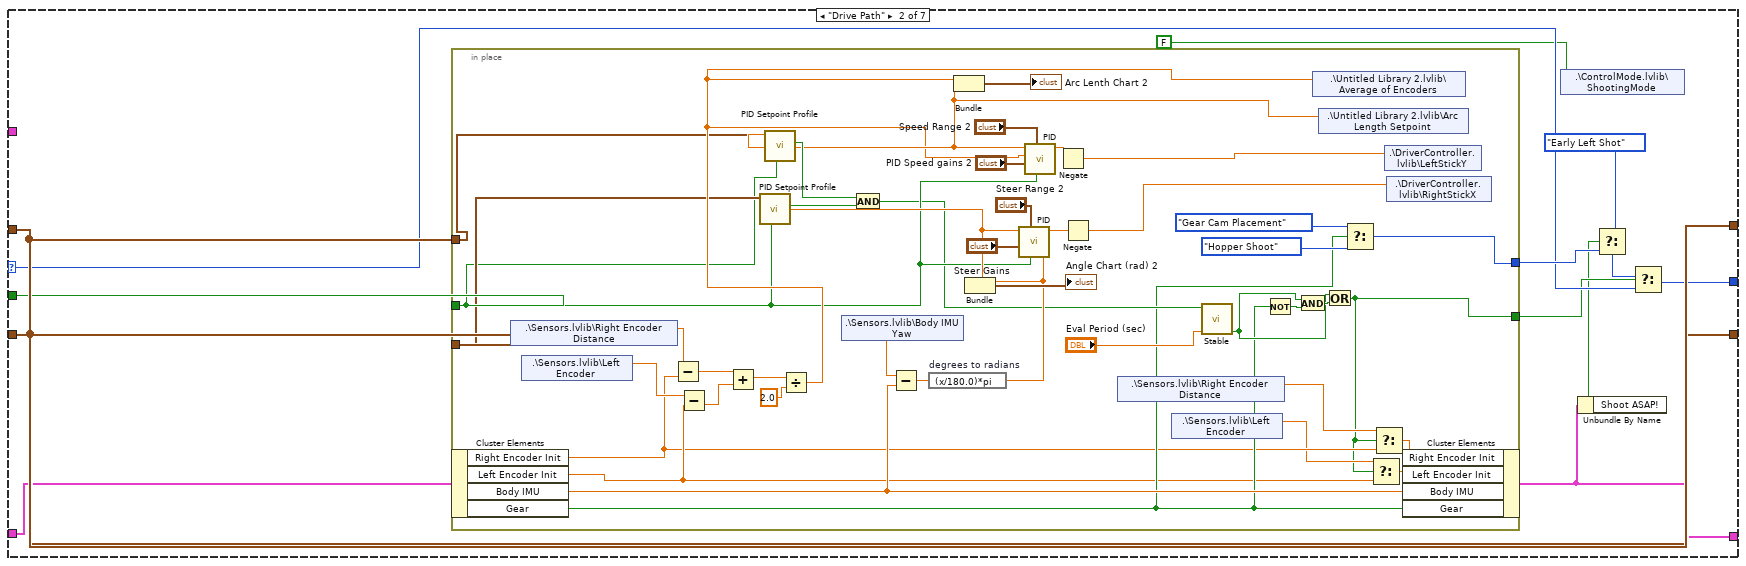
[diagram p10: hidden frame]
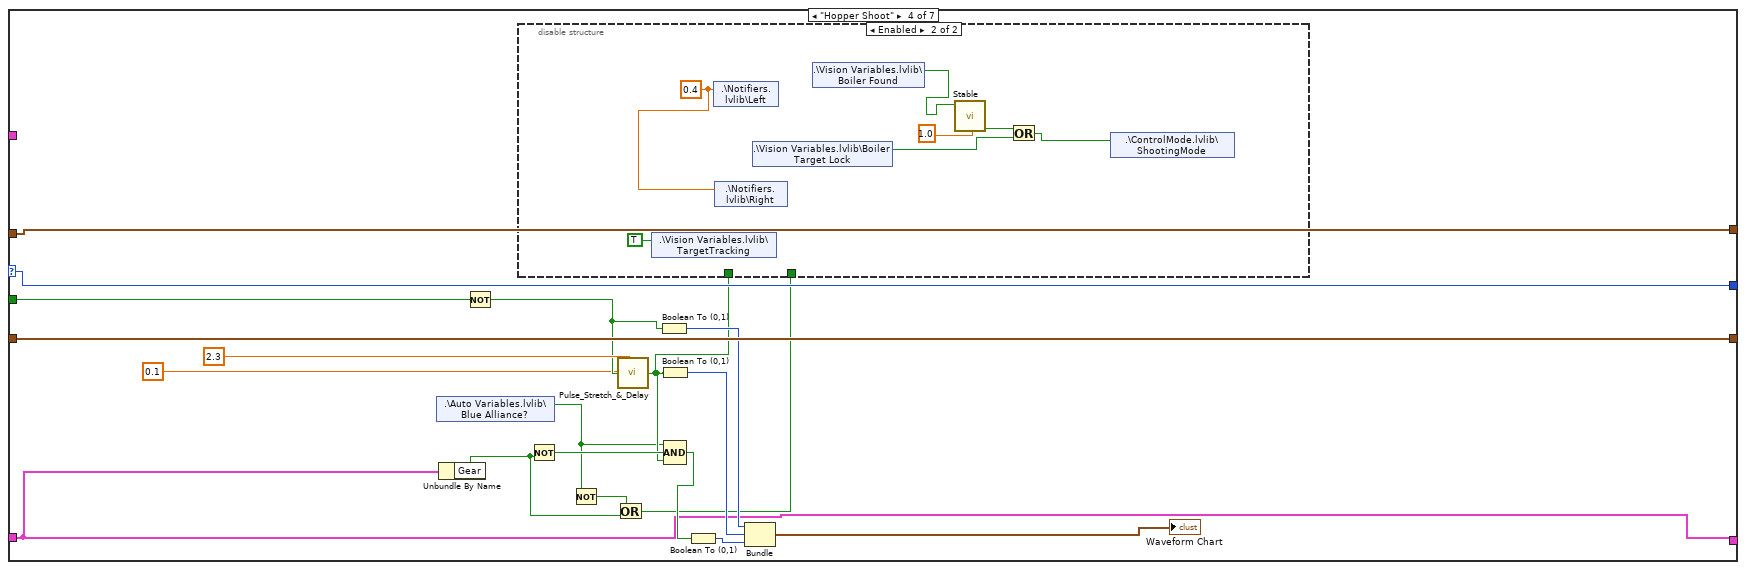
[diagram p15: hidden frame]
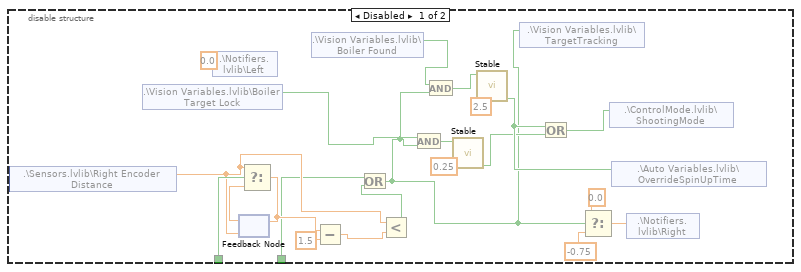
[diagram p16: hidden frame]
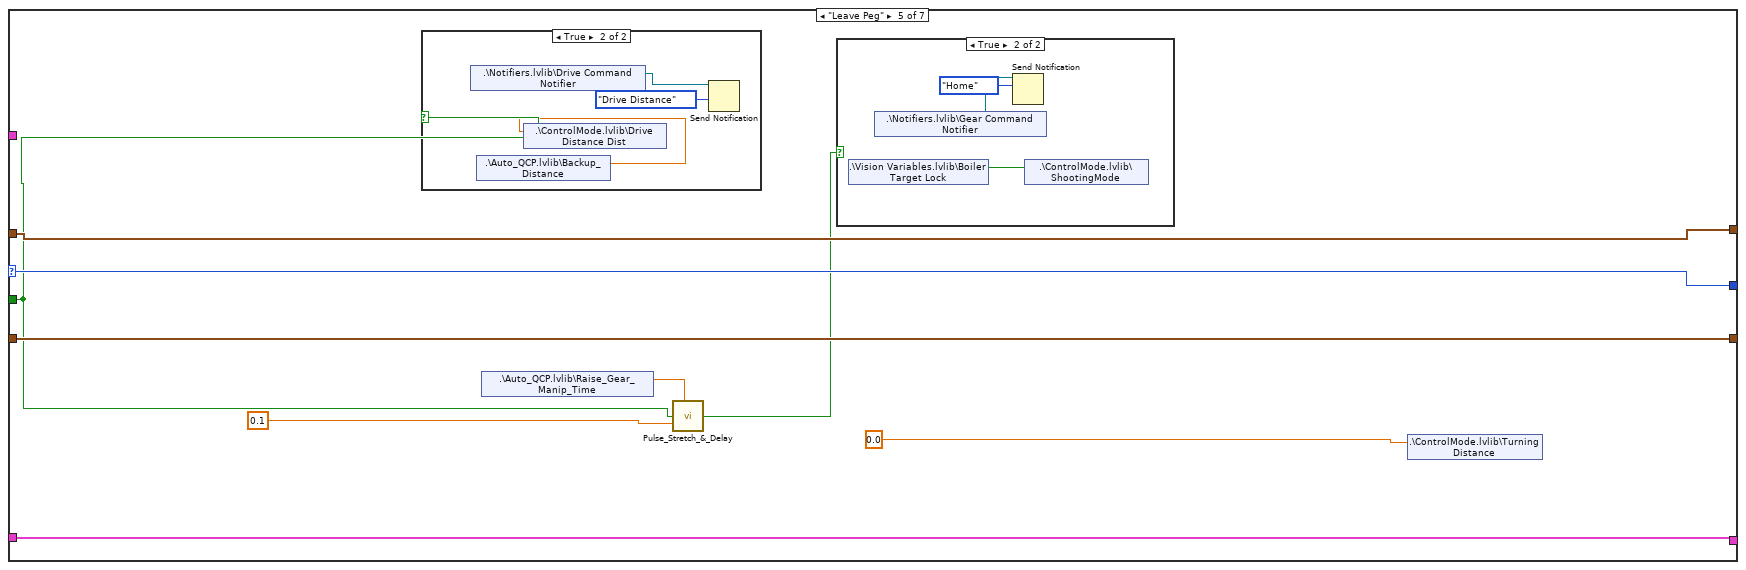
[diagram p17: hidden frame]
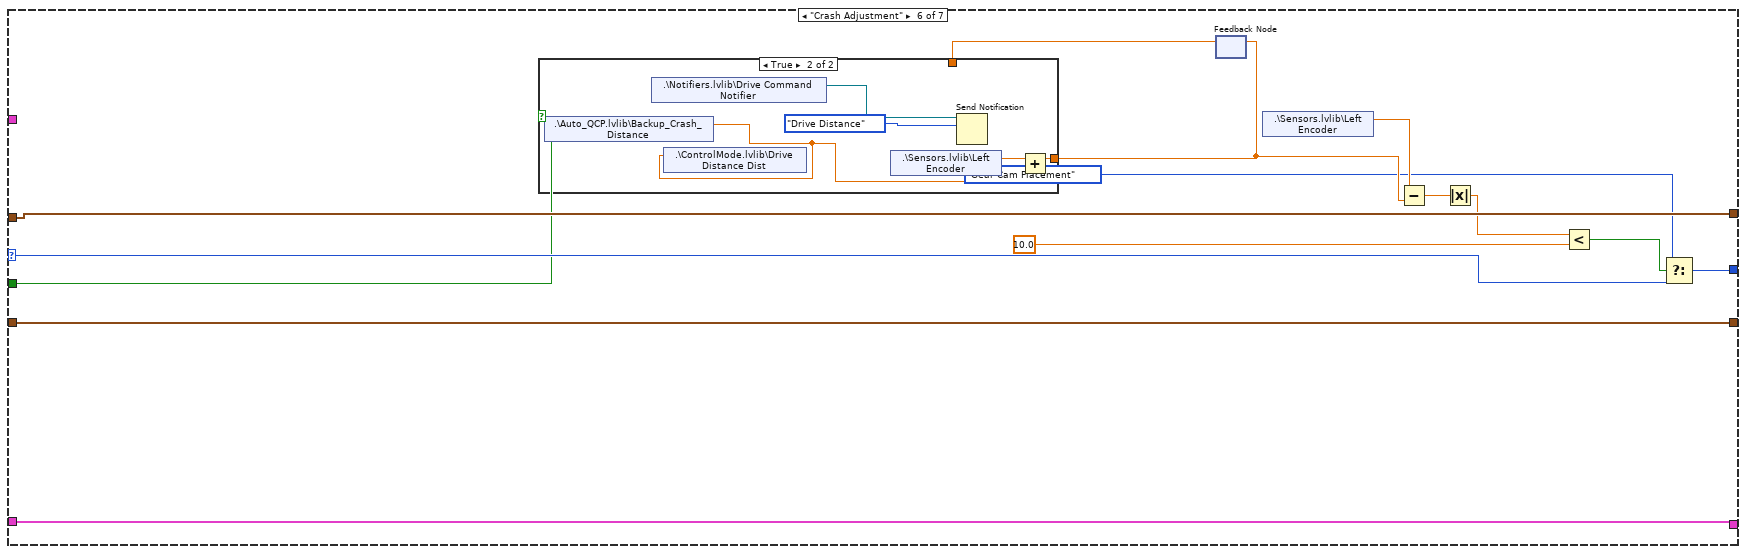
[diagram p20: hidden frame]
diagram:
  (unwired) T5 {"X"=[0.0, 26.60027335008321, 40.72548065744226], "Y"=[0.0, 13.070920440908349, 15.27217301482698], "Absolute Theta initial"=0.0, "Absolute Theta final"=0.0}
  w19 = cluster{dbl, dbl}[] []
  w13 = AutoStates."Calculate Path"
  # "TEMPORARY\nNeeds QCP"
  # "Initial\nValues"
  # "Theta"
  # "S"
  n1 = call-poly <vilib>:"NT Read Value.vi"("Default Value"=4.0, "Name"="Path Time") -> ("Numeric"=w9:dbl)  [unwired: 8 in, 1 out]
  n2 = call-poly <vilib>:"NT Read Value.vi"("Default Value"=0.0, "Name"="Offset") -> ("Numeric"=w4:dbl)  [unwired: 8 in, 1 out]
  n3 = call-poly <vilib>:"NT Read Value.vi"("Default Value"=TRUE, "Name"="Gear?") -> ("Boolean"=w15:bool)  [unwired: 8 in, 1 out]
  n4 = call-poly <vilib>:"NT Read Value.vi"("Default Value"=FALSE, "Name"="Shoot ASAP!") -> ("Boolean"=w5:bool)  [unwired: 8 in, 1 out]
  n5 = shared-variable ".\\Auto Variables.lvlib\\Blue Alliance?"() -> (w14:bool)  [unwired: 1 in, 1 out]
  n6 = case shown="True" w15 {
    tunnel: [w66 w79] -> w18
    tunnel: w14 -> [w69 w72]
    tunnel: [GearPositions."Left" w81] -> w12
    tunnel: w9 -> [w64 _]
    tunnel: w4 -> [w33 w78]
    tunnel: w5 -> [_ w77]
    frame False {
      # "far hopper"
      # "0 110 133"
      # "0 0 -40"
      # "close hopper"
      # "0 67 82"
      # "0 0 -42"
      n7 = shared-variable ".\\Auto_QCP.lvlib\\Hopper_Theta_Initial"() -> (w48:dbl)  [unwired: 1 in, 1 out]
      n8 = shared-variable ".\\Auto_QCP.lvlib\\Hopper_Theta_Final"() -> (w47:dbl)  [unwired: 1 in, 1 out]
      n9 = shared-variable ".\\Auto_QCP.lvlib\\Hopper_Time_Taken"() -> (w46:dbl)  [unwired: 1 in, 1 out]
      n10 = shared-variable ".\\Auto_QCP.lvlib\\Close_Hopper_Y"() -> (w49:dbl[])  [unwired: 1 in, 1 out]
      n11 = shared-variable ".\\Auto_QCP.lvlib\\Close_Hopper_X"() -> (w50:dbl[])  [unwired: 1 in, 1 out]
      n12 = call-poly <vilib>:"NT Read Value.vi"("Name"="Far Hopper?") -> ("Boolean"=w38:bool)  [unwired: 9 in, 1 out]
      n13 = Multiply(x=w33, y=0.25) -> (x*y=w31:dbl)
      n14 = Bundle By Name(cluster=T1 {"X"=[0.0, 0.0, -42.0], "Y"=[0.0, 71.0, 91.0], "Absolute Theta initial"=1.570796, "Absolute Theta final"=3.14159, "Amount of Time (s) 2"=3.5} ("Drive Path Control"), "X"=w50, "Y"=w49, "Absolute Theta initial"=w48, "Absolute Theta final"=w47, "Amount of Time (s) 2"=w46) -> (w51:T1)
      n15 = Build Array(w33, w31, -44.0 ("t")) -> (w65:dbl[])
      n16 = shared-variable ".\\Auto_QCP.lvlib\\Hopper_Trigger_Y_Offset"() -> (w44:dbl[])  [unwired: 1 in, 1 out]
      n17 = shared-variable ".\\Auto_QCP.lvlib\\Far_Hopper_Y_Offset"() -> (w45:dbl[])  [unwired: 1 in, 1 out]
      n18 = Unbundle By Name(w51) -> ("Y"=w63:dbl[])
      n19 = call-poly <vilib>:"NT Read Value.vi"("Name"="Trigger?") -> ("Boolean"=w53:bool)  [unwired: 9 in, 1 out]
      n20 = Add(x=w63, y=w45) -> (x+y=w62:dbl[])
      n21 = Negate(x=w44) -> (-x=w60:dbl[])
      n22 = Select(t=w62, s=w38, f=w63) -> (s? t:f=w57:dbl[])
      n23 = Select(t=w44, s=w38, f=w60) -> (s? t:f=w59:dbl[])
      n24 = Add(x=w57, y=w59) -> (x+y=w58:dbl[])
      n25 = Select(t=w57, s=w53, f=w58) -> (s? t:f=w56:dbl[])
      n26 = Bundle By Name(cluster=w51, "X"=w65, "Y"=w56, "Amount of Time (s) 2"=w64) -> (w66:T1)
      n27 = shared-variable ".\\Auto_QCP.lvlib\\Hopper_Red_Turret"() -> (w43:dbl)  [unwired: 1 in, 1 out]
      n28 = shared-variable ".\\Auto_QCP.lvlib\\Hopper_Blue_Turret"() -> (w42:dbl)  [unwired: 1 in, 1 out]
      n29 = Select(t=1630.0, s=w38, f=1732.0) -> (s? t:f=w39:dbl)
      n30 = Select(t=-6075.0, s=w38, f=-4212.0) -> (s? t:f=w40:dbl)
      n31 = shared-variable ".\\ControlMode.lvlib\\Fixed RPM Mode"(TRUE ("Fixed RPM Mode")) -> ()  [unwired: 1 in, 1 out]
      n32 = shared-variable ".\\Vision Variables.lvlib\\TargetTracking"(FALSE ("TargetTracking")) -> ()  [unwired: 1 in, 1 out]
      n33 = shared-variable ".\\ControlMode.lvlib\\FixedBottomRPM"(w39) -> ()  [unwired: 1 in, 1 out]
      n34 = shared-variable ".\\ControlMode.lvlib\\Fixed Top RPM"(w40) -> ()  [unwired: 1 in, 1 out]
      n35 = Select(t=w42, s=w69, f=w43) -> (s? t:f=w68:dbl)
      n36 = shared-variable ".\\Vision Variables.lvlib\\TurretDesiredAngle"(w68) -> ()  [unwired: 1 in, 1 out]
    }
    frame True {
      n37 = shared-variable ".\\Auto Variables.lvlib\\Blue Alliance?"() -> (w84:bool)  [unwired: 1 in, 1 out]
      n38 = call-poly <vilib>:"NT Read Value.vi"("Name"="Peg") -> ()  [unwired: 9 in, 2 out]
      n39 = To Unsigned Word Integer(number=u16 0) -> (unsigned 16bit integer=w82:u16)
      n40 = Type Cast(type=GearPositions."Left", x=w82) -> (*(type *) &x=w83:T3)
      n41 = case shown="False" w84 {
        tunnel: w83 -> [w95 w101]
        tunnel: [w99 w101] -> w81
        frame False {
          w96 = GearPositions."Right" ("t")
          w98 = GearPositions."Left" ("t")
          n42 = Equal?(x=w98, y=w95) -> (x = y?=w97:bool)
          n43 = Equal?(x=w95, y=w96) -> (x = y?=w94:bool)
          n44 = Select(t=w96, s=w97, f=w95) -> (s? t:f=w100:T3)
          n45 = Select(t=w98, s=w94, f=w100) -> (s? t:f=w99:T3)
        }
        frame True {
        }
      }
      n46 = case shown="\"Right\"" w81 {
        tunnel: [w107 w114 w116] -> w80
        frame "Left", Default {
          # "0.5016"
          # "Blue:\nLeft PEG"
          n47 = shared-variable ".\\Auto_QCP.lvlib\\Left_Peg_Theta_Init"() -> (w102:dbl)  [unwired: 1 in, 1 out]
          n48 = shared-variable ".\\Auto_QCP.lvlib\\Left_Peg_Theta_Final"() -> (w106:dbl)  [unwired: 1 in, 1 out]
          n49 = shared-variable ".\\Auto_QCP.lvlib\\Left_Peg_X"() -> (w104:dbl[])  [unwired: 1 in, 1 out]
          n50 = shared-variable ".\\Auto_QCP.lvlib\\Left_Peg_Y"() -> (w103:dbl[])  [unwired: 1 in, 1 out]
          n51 = shared-variable ".\\Auto_QCP.lvlib\\Left_Peg_Time_Taken"() -> (w105:dbl)  [unwired: 1 in, 1 out]
          n52 = Bundle By Name(cluster=T1 {"X"=[0.0, 26.0], "Y"=[0.0, 91.0], "Absolute Theta initial"=1.570796, "Absolute Theta final"=0.54, "Amount of Time (s) 2"=3.5} ("Drive Path Control"), "X"=w104, "Y"=w103, "Absolute Theta initial"=w102, "Absolute Theta final"=w106, "Amount of Time (s) 2"=w105) -> (w107:T1)
        }
        frame "Center" {
          # "Blue:\nCenter PEG"
          n53 = shared-variable ".\\Auto_QCP.lvlib\\Center_Peg_Y"() -> (w112:dbl[])  [unwired: 1 in, 1 out]
          n54 = shared-variable ".\\Auto_QCP.lvlib\\Ceter_Peg_Theta_Init"() -> (w111:dbl)  [unwired: 1 in, 1 out]
          n55 = shared-variable ".\\Auto_QCP.lvlib\\Center_Peg_X"() -> (w113:dbl[])  [unwired: 1 in, 1 out]
          n56 = shared-variable ".\\Auto_QCP.lvlib\\Center_Peg_Theta_Final"() -> (w110:dbl)  [unwired: 1 in, 1 out]
          n57 = shared-variable ".\\Auto_QCP.lvlib\\Center_Peg_Time_Taken"() -> (w109:dbl)  [unwired: 1 in, 1 out]
          n58 = Bundle By Name(cluster=T1 {"X"=[112.0, 112.0], "Y"=[0.0, 35.0], "Absolute Theta initial"=1.570796, "Absolute Theta final"=1.5708, "Amount of Time (s) 2"=1.0} ("Drive Path Control"), "X"=w113, "Y"=w112, "Absolute Theta initial"=w111, "Absolute Theta final"=w110, "Amount of Time (s) 2"=w109) -> (w114:T1)
        }
        frame "Right" {
          w116 = T1 {"X"=[214.0, 188.0], "Y"=[0.0, 93.0], "Absolute Theta initial"=1.570796, "Absolute Theta final"=2.5, "Amount of Time (s) 2"=3.5} ("Drive Path Control")
          # "Blue:\nRIGHT GEAR PEG"
          n59 = shared-variable ".\\Auto_QCP.lvlib\\Right_Peg_Time_Taken"() -> (w117:dbl)  [unwired: 1 in, 1 out]
          n60 = shared-variable ".\\Auto_QCP.lvlib\\Right_Peg_X"() -> (w121:dbl[])  [unwired: 1 in, 1 out]
          n61 = shared-variable ".\\Auto_QCP.lvlib\\Right_Peg_Y"() -> (w120:dbl[])  [unwired: 1 in, 1 out]
          n62 = shared-variable ".\\Auto_QCP.lvlib\\Right_Peg_Thata_Init"() -> (w119:dbl)  [unwired: 1 in, 1 out]
          n63 = shared-variable ".\\Auto_QCP.lvlib\\Right_Peg_Theta_Final"() -> (w118:dbl)  [unwired: 1 in, 1 out]
          n64 = Bundle By Name(cluster=w116, "X"=w121, "Y"=w120, "Absolute Theta initial"=w119, "Absolute Theta final"=w118, "Amount of Time (s) 2"=w117) -> ()  [unwired: 1 out]
        }
      }
      n65 = shared-variable ".\\Auto_QCP.lvlib\\Hopper_Red_Turret"() -> (w74:dbl)  [unwired: 1 in, 1 out]
      n66 = Not(x=w77) -> (.not. x?=w76:bool)
      n67 = shared-variable ".\\Auto_QCP.lvlib\\Hopper_Blue_Turret"() -> (w73:dbl)  [unwired: 1 in, 1 out]
      n68 = in-place {
        in-place-border: w78 -> [w90]
        n69 = in-place-cluster #1(w80) -> ("X"=w89:dbl[])
        n70 = in-place {
          in-place-border: w90 -> [w93]
          n71 = in-place-array #2(w89, 0) -> (w92:dbl)
          n72 = Add(x=w92, y=w93) -> (x+y=w91:dbl)
          n73 = in-place-array #2(w91) -> (w88:dbl[])  [unwired: 1 out]
        }
        n74 = in-place-cluster #1("X"=w88) -> (w79:T1)
      }
      n75 = shared-variable ".\\Vision Variables.lvlib\\TargetTracking"(w76) -> ()  [unwired: 1 in, 1 out]
      n76 = Select(t=w73, s=w72, f=w74) -> (s? t:f=w75:dbl)
      n77 = shared-variable ".\\Vision Variables.lvlib\\TurretDesiredAngle"(w75) -> ()  [unwired: 1 in, 1 out]
    }
  }
  n78 = shared-variable ".\\Sensors.lvlib\\Right Encoder Distance"() -> (w20:dbl)  [unwired: 1 in, 1 out]
  n79 = case shown="False" w14 {
    tunnel: w18 -> [w129 w132]
    tunnel: [w122 w132] -> w17
    frame False {
      n80 = Unbundle By Name(w129) -> ("Absolute Theta initial"=w125:dbl)
      n81 = Unbundle By Name(w129) -> ("Absolute Theta final"=w128:dbl)
      n82 = Unbundle By Name(w129) -> ("X"=w131:dbl[])
      n83 = Negate(x=w131) -> (-x=w130:dbl[])
      n84 = Subtract(x=w128, y=w125) -> (x-y=w127:dbl)
      n85 = Bundle By Name(cluster=w129, "X"=w130) -> (w123:T1)
      n86 = Negate(x=w127) -> (-x=w126:dbl)
      n87 = Add(x=w126, y=w125) -> (x+y=w124:dbl)
      n88 = Bundle By Name(cluster=w123, "Absolute Theta final"=w124) -> (w122:T1)
    }
    frame True {
    }
  }
  n89 = shared-variable ".\\Sensors.lvlib\\Body IMU Yaw"() -> (w25:dbl)  [unwired: 1 in, 1 out]
  n90 = shared-variable ".\\Sensors.lvlib\\Left Encoder"() -> (w21:dbl)  [unwired: 1 in, 1 out]
  n91 = Tick Count (ms)() -> (millisecond timer value=w11:u32)
  n92 = Unbundle By Name(w17) -> ("Absolute Theta initial"=w27:dbl)
  n93 = expression code="(x/pi)*180.0" "radians to degrees"(w27) -> (w28:dbl)
  n94 = Subtract(x=w25, y=w28) -> (x-y=w26:dbl)
  n95 = Bundle(cluster=T4 {"Body IMU"=0.0, "Right Encoder Init"=0.0, "Left Encoder Init"=0.0, "Gear"=TRUE, "Peg"=enum."Left", "Initial Time"=0, "Shoot ASAP!"=FALSE}, "Body IMU"=w26, "Right Encoder Init"=w20, "Left Encoder Init"=w21, "Gear"=w15, "Peg"=w12, "Initial Time"=w11, "Shoot ASAP!"=w5) -> (w22:T4)
  n96 = node-c288(i64 50 ("Period")) -> (w30:T7)  [unwired: 3 in]
  n97 = timed-loop {
    timing: w30 -> [_]
    timing-out: [_] -> w29
    shift-right: [w143] -> _
    shift-left: w13 -> [w137]
    shift-right: [w142] -> _
    shift-left: w19 -> [w140]
    shift-right: [w141] -> _
    shift-left: w19 -> [w139]
    shift-left: w13 -> [w136]
    tunnel: w17 -> [w134]
    shift-right: [w133] -> _
    shift-left: w22 -> [w138]
    stop <- FALSE stop-if-true
    n98 = node-c288() -> ()  [unwired: 1 in, 1 out]
    n99 = shared-variable ".\\ToLog.lvlib\\Auto State"(w137) -> ()  [unwired: 1 in, 1 out]
    n100 = Not Equal?(x=w137, y=w136) -> (x != y?=w135:bool)
    n101 = case shown="\"Gear Cam Placement\"" w137 {
      selector: w137 -> [_ w232 w290 w352 w390 w409 w433]
      tunnel: [w187 w234 w286 w352 w390 w408 w434] -> w143
      tunnel: [w200 w238 w292 w354 w392 w411 w437] -> w142
      tunnel: [w199 w237 w291 w353 w391 w412 w436] -> w141
      tunnel: w140 -> [_ w238 w292 w354 w392 w411 w437]
      tunnel: w139 -> [_ w237 w291 w353 w391 w412 w436]
      tunnel: w138 -> [w167 w235 w288 w336 w386 w410 w435]
      tunnel: w135 -> [_ w236 w289 w345 w388 w407 w425]
      tunnel: w134 -> [w198 _ _ _ _ _ _]
      tunnel: [w170 w229 w287 w336 w386 w410 w435] -> w133
      frame "Calculate Path", Default {
        n102 = First Call?() -> (First Call?: T/F=w159:bool)
        n103 = Unbundle By Name(w167) -> ("Shoot ASAP!"=w147:bool, "Gear"=w145:bool)
        n104 = Not(x=w159) -> (.not. x?=w162:bool)
        n105 = Not(x=w147) -> (.not. x?=w146:bool)
        n106 = shared-variable ".\\Auto_QCP.lvlib\\Orient_Change_Limit"() -> (w183:dbl)  [unwired: 1 in, 1 out]
        n107 = call <userlib>:"Stable.vi"("Eval Period (sec)"=0.4, "Signal Input"=w162) -> ("Stable"=w160:bool)  [unwired: 9 in]
        n108 = Unbundle By Name(w198) -> ("X"=w179:dbl[], "Y"=w197:dbl[], "Absolute Theta initial"=w196:dbl, "Absolute Theta final"=w195:dbl, "Amount of Time (s) 2"=w194:dbl)
        n109 = And(x=w146, y=w145) -> (x .and. y?=w148:bool)
        n110 = Index Array(array=w179, index=0) -> (element=w177:dbl)
        n111 = Absolute Value(x=w177) -> (abs(x)=w168:dbl)
        n112 = Greater?(x=w168, y=20.0) -> (0:w152:bool)
        n113 = And(x=w147, y=w152) -> (x .and. y?=w154:bool)
        n114 = And(x=w160, y=w154) -> (x .and. y?=w153:bool)
        n115 = Or(x=w153, y=w148) -> (x .or. y?=w149:bool)
        n116 = shared-variable ".\\Vision Variables.lvlib\\TargetTracking"(w149) -> ()  [unwired: 1 in, 1 out]
        n117 = Not(x=w154) -> (.not. x?=w169:bool)
        n118 = Not(x=w152) -> (.not. x?=w151:bool)
        n119 = And(x=w169, y=w147) -> (x .and. y?=w166:bool)
        n120 = And(x=w151, y=w145) -> (x .and. y?=w150:bool)
        n121 = call "ArcAndTheta.vi"("Limit of Orientation Change"=w183, "Amount of Time (s)"=w194, "Absolute Theta Final"=w195, "Absolute Theta initial"=w196, "Y"=w197, "X"=w179) -> ("Theta(arc length)"=w206:dbl[], "Arc Length"=w207:dbl[], "TimeStamp"=w205:dbl[], "Verify Graph"=→"Verify Graph 2":cluster{"X":dbl, "Y":dbl}[])  [unwired: 2 in]
        n122 = case shown="True" w150 {
          frame False {
          }
          frame True {
            n123 = shared-variable ".\\Vision Variables.lvlib\\TurretDesiredAngle"(-15.0 ("TurretDesiredAngle")) -> ()  [unwired: 1 in, 1 out]
          }
        }
        n124 = shared-variable ".\\Auto_QCP.lvlib\\Pid_Segments"() -> (w182:dbl)  [unwired: 1 in, 1 out]
        n125 = call-poly <vilib>:"NT Read Value.vi"("Name"="Delay") -> ("Numeric"=w185:dbl)  [unwired: 9 in, 1 out]
        n126 = Build Cluster Array(w205, w207) -> (w203:cluster{dbl, dbl}[])
        n127 = Build Cluster Array(w205, w206) -> (w202:cluster{dbl, dbl}[])
        n128 = call <userlib>:"Pulse_Stretch_&_Delay.vi"("Delay (sec)"=1.0, "In"=w153, "Width (sec)"=3.0) -> ("Out"=w155:bool)  [unwired: 2 in]
        n129 = Array Size(array=w205) -> (size(s)=w204:i32)
        n130 = shared-variable ".\\Vision Variables.lvlib\\Boiler Target Lock"() -> (w164:bool)  [unwired: 1 in, 1 out]
        n131 = for {
          N: w182 -> [w225]
          tunnel: w204 -> [w223]
          tunnel: w203 -> [w217]
          tunnel: w202 -> [w216]
          tunnel: [w214] -> w200 mode=indexing
          tunnel: [w213] -> w199 mode=indexing
          i -> [w221]
          n132 = Reciprocal(x=w225) -> (1/x=w224:dbl)
          n133 = Increment(x=w221) -> (x+1=w220:i32)
          n134 = Multiply(x=w224, y=w223) -> (x*y=w222:dbl)
          n135 = Round Toward -Infinity(1:w222) -> (0:w219:dbl)
          n136 = Multiply(x=w219, y=w220) -> (x*y=w218:dbl)
          n137 = Decrement(x=w218) -> (x-1=w215:dbl)
          n138 = Index Array(array=w217, index=w215) -> (element=w214:cluster{dbl, dbl})
          n139 = Index Array(array=w216, index=w215) -> (element=w213:cluster{dbl, dbl})
        }
        n140 = Unbundle By Name(w167) -> ("Initial Time"=w192:u32)
        n141 = Tick Count (ms)() -> (millisecond timer value=w193:u32)
        n142 = And(x=w153, y=w164) -> (x .and. y?=w163:bool)
        n143 = Or(x=w163, y=w155) -> (x .or. y?=w158:bool)
        n144 = Subtract(x=w193, y=w192) -> (x-y=w181:u32)
        n145 = shared-variable ".\\ControlMode.lvlib\\ShootingMode"(w158) -> ()  [unwired: 1 in, 1 out]
        n146 = To Double Precision Float(number=w181) -> (double precision float=w184:dbl)
        n147 = Greater?(x=w181, y=u32 5500) -> (0:w175:bool)
        n148 = Multiply(x=w185, y=1000.0) -> (x*y=w191:dbl)
        n149 = Greater?(x=w184, y=w191) -> (0:w173:bool)
        n150 = Not(x=w154) -> (.not. x?=w172:bool)
        n151 = Compound Arithmetic op=AND(w154, w175, w173) -> (w174:bool)
        n152 = And(x=w172, y=w173) -> (x .and. y?=w171:bool)
        n153 = Or(x=w174, y=w171) -> (x .or. y?=w165:bool)
        n154 = case shown="True" w165 {
          tunnel: [w209 w212] -> w170
          tunnel: w167 -> [w209 w211]
          tunnel: w166 -> [_ w210]
          frame False {
          }
          frame True {
            n155 = Bundle By Name(cluster=w211, "Shoot ASAP!"=w210) -> (w212:T4)
          }
        }
        n156 = Select(t=AutoStates."Drive Path", s=w165, f=AutoStates."Calculate Path") -> (s? t:f=w187:T6)
      }
      frame "Drive Path" {
        n157 = in-place {
          in-place-border: w238 -> [w258]
          in-place-border: w237 -> [w257]
          in-place-border: w236 -> [w254]
          in-place-border: [w240] -> w233
          in-place-border: [w239] -> w230
          n158 = in-place-cluster #3(w235) -> ("Right Encoder Init"=w243:dbl, "Left Encoder Init"=w244:dbl, "Body IMU"=w248:dbl, "Gear"=w247:bool)
          n159 = shared-variable ".\\Sensors.lvlib\\Right Encoder Distance"() -> (w270:dbl)  [unwired: 1 in, 1 out]
          n160 = shared-variable ".\\Sensors.lvlib\\Left Encoder"() -> (w272:dbl)  [unwired: 1 in, 1 out]
          n161 = Subtract(x=w270, y=w243) -> (x-y=w269:dbl)
          n162 = Subtract(x=w272, y=w244) -> (x-y=w271:dbl)
          n163 = Add(x=w269, y=w271) -> (x+y=w277:dbl)
          n164 = call <vilib>:"PID Setpoint Profile.vi"("reinitialize? (F)"=w254, "setpoint profile"=w257) -> ("profile complete?"=w281:bool, "setpoint"=w279:dbl)  [unwired: 4 in, 2 out]
          n165 = call <vilib>:"PID Setpoint Profile.vi"("reinitialize? (F)"=w254, "setpoint profile"=w258) -> ("profile complete?"=w280:bool, "setpoint"=w266:dbl)  [unwired: 4 in, 2 out]
          n166 = Divide(x=w277, y=2.0) -> (x/y=w260:dbl)
          n167 = shared-variable ".\\Sensors.lvlib\\Body IMU Yaw"() -> (w265:dbl)  [unwired: 1 in, 1 out]
          n168 = And(x=w280, y=w281) -> (x .and. y?=w252:bool)
          n169 = Subtract(x=w265, y=w248) -> (x-y=w256:dbl)
          n170 = expression code="(x/180.0)*pi" "degrees to radians"(w256) -> (w255:dbl)
          n171 = Bundle(w260, "setpoint"=w266) -> (→"Arc Lenth Chart 2":cluster{dbl, "setpoint":dbl})  [unwired: 1 in]
          n172 = Bundle(w255, "setpoint"=w279) -> (→"Angle Chart (rad) 2":cluster{dbl, "setpoint":dbl})  [unwired: 1 in]
          n173 = call-poly <vilib>:"PID.vi"("reinitialize? (F)"=w254, "output range"="Steer Range 2", "PID gains"="Steer Gains", "process variable"=w255, "setpoint"=w279) -> ("output"=w267:dbl)  [unwired: 5 in, 1 out]
          n174 = call-poly <vilib>:"PID.vi"("reinitialize? (F)"=w254, "output range"="Speed Range 2", "PID gains"="PID Speed gains 2", "process variable"=w260, "setpoint"=w266) -> ("output"=w268:dbl)  [unwired: 5 in, 1 out]
          n175 = Negate(x=w268) -> (-x=w263:dbl)
          n176 = Negate(x=w267) -> (-x=w262:dbl)
          n177 = shared-variable ".\\Sensors.lvlib\\Right Encoder Distance"() -> (w242:dbl)  [unwired: 1 in, 1 out]
          n178 = shared-variable ".\\Sensors.lvlib\\Left Encoder"() -> (w241:dbl)  [unwired: 1 in, 1 out]
          n179 = call <userlib>:"Stable.vi"("Eval Period (sec)"="Eval Period (sec)", "Signal Input"=w252) -> ("Stable"=w249:bool)  [unwired: 9 in]
          n180 = Not(x=w247) -> (.not. x?=w250:bool)
          n181 = And(x=w249, y=w250) -> (x .and. y?=w251:bool)
          n182 = shared-variable ".\\Untitled Library 2.lvlib\\Average of Encoders"(w260) -> ()  [unwired: 1 in, 1 out]
          n183 = shared-variable ".\\Untitled Library 2.lvlib\\Arc Length Setpoint"(w266) -> ()  [unwired: 1 in, 1 out]
          n184 = Or(x=w249, y=w251) -> (x .or. y?=w239:bool)
          n185 = Select(t=AutoStates."Gear Cam Placement", s=w247, f=AutoStates."Hopper Shoot") -> (s? t:f=w240:T6)
          n186 = Select(t=w241, s=w239, f=w244) -> (s? t:f=w245:dbl)
          n187 = Select(t=w242, s=w239, f=w243) -> (s? t:f=w246:dbl)
          n188 = shared-variable ".\\DriverController.lvlib\\LeftStickY"(w263) -> ()  [unwired: 1 in, 1 out]
          n189 = shared-variable ".\\DriverController.lvlib\\RightStickX"(w262) -> ()  [unwired: 1 in, 1 out]
          n190 = in-place-cluster #3("Right Encoder Init"=w246, "Left Encoder Init"=w245, "Body IMU"=w248, "Gear"=w247) -> (w229:T4)
        }
        n191 = shared-variable ".\\ControlMode.lvlib\\ShootingMode"(FALSE ("ShootingMode")) -> ()  [unwired: 1 in, 1 out]
        n192 = Unbundle By Name(w229) -> ("Shoot ASAP!"=w228:bool)
        n193 = Select(t=AutoStates."Early Left Shot", s=w228, f=w233) -> (s? t:f=w231:T6)
        n194 = Select(t=w231, s=w230, f=w232) -> (s? t:f=w234:T6)
      }
      frame "Gear Cam Placement" {
        n195 = flat-sequence {
          tunnel: w288 -> [w294]
          tunnel: w289 -> [w293]
          tunnel: w290 -> [w295]
          tunnel: [w295] -> w285
          tunnel: [w293] -> w284
          tunnel: [w294] -> w283
          tunnel: [w307] -> w287
          tunnel: [w300] -> w286
          tunnel: w285 -> [w322]
          tunnel: w284 -> [w309]
          tunnel: w283 -> [w308]
          frame #0 {
            n196 = case shown="True" w293 {
              frame False {
              }
              frame True {
                w296 = 0.0
                n197 = shared-variable ".\\DriverController.lvlib\\LeftStickY"(w296) -> ()  [unwired: 1 in, 1 out]
                n198 = shared-variable ".\\DriverController.lvlib\\RightStickX"(w296) -> ()  [unwired: 1 in, 1 out]
              }
            }
          }
          frame #1 {
            n199 = shared-variable ".\\Vision Variables.lvlib\\Gear valid"() -> (w315:bool)  [unwired: 1 in, 1 out]
            n200 = shared-variable ".\\Auto_QCP.lvlib\\Gear_Place_Timeout"() -> (w297:dbl)  [unwired: 1 in, 1 out]
            n201 = feedback #4() -> (w318:bool)  [unwired: 1 in]
            n202 = feedback-in #4(w315) -> ()
            n203 = Not(x=w315) -> (.not. x?=w316:bool)
            n204 = And(x=w316, y=w309) -> (x .and. y?=w312:bool)
            n205 = case shown="True" w312 {
              frame False {
              }
              frame True {
                n206 = shared-variable ".\\Auto_QCP.lvlib\\Failsafe_Distance"() -> (w324:dbl)  [unwired: 1 in, 1 out]
                n207 = shared-variable ".\\Notifiers.lvlib\\Drive Command Notifier"() -> (w326:refnum<notifier>)  [unwired: 1 in, 1 out]
                n208 = shared-variable ".\\ControlMode.lvlib\\Drive Distance Dist"(w324) -> ()  [unwired: 1 in, 1 out]
                n209 = Send Notification(notification=Drive_Commands."Drive Distance", notifier=w326) -> ()  [unwired: 1 in, 2 out]
              }
            }
            n210 = And(x=w309, y=w315) -> (x .and. y?=w314:bool)
            n211 = call <userlib>:"Pulse_Stretch_&_Delay.vi"("Delay (sec)"=w297, "In"=w309, "Width (sec)"=0.1) -> ("Out"=w301:bool)  [unwired: 2 in]
            n212 = Greater?(x=w315, y=w318) -> (0:w317:bool)
            n213 = Or(x=w317, y=w314) -> (x .or. y?=w313:bool)
            n214 = case shown="True" w313 {
              frame False {
              }
              frame True {
                n215 = shared-variable ".\\Notifiers.lvlib\\Drive Command Notifier"() -> (w330:refnum<notifier>)  [unwired: 1 in, 1 out]
                n216 = shared-variable ".\\DriverController.lvlib\\RightStickX"(0.0 ("LeftStickY")) -> ()  [unwired: 1 in, 1 out]
                n217 = shared-variable ".\\DriverController.lvlib\\LeftStickY"(-1.0 ("LeftStickY")) -> ()  [unwired: 1 in, 1 out]
                n218 = Send Notification(notification=Drive_Commands."Place Gear", notifier=w330) -> ()  [unwired: 1 in, 2 out]
              }
            }
            n219 = shared-variable ".\\Sensors.lvlib\\Left Encoder"() -> (w304:dbl)  [unwired: 1 in, 1 out]
            n220 = shared-variable ".\\Sensors.lvlib\\Gear Distance Within Tol"() -> (w323:bool)  [unwired: 1 in, 1 out]
            n221 = shared-variable ".\\Sensors.lvlib\\Gear Overdoned"() -> (w299:bool)  [unwired: 1 in, 1 out]
            n222 = shared-variable ".\\Auto_QCP.lvlib\\After_Spline_Cutoff_Dist"() -> (w302:dbl)  [unwired: 1 in, 1 out]
            n223 = Unbundle By Name(w308) -> ("Left Encoder Init"=w305:dbl)
            n224 = Subtract(x=w304, y=w305) -> (x-y=w311:dbl)
            n225 = Greater?(x=w311, y=w302) -> (0:w310:bool)
            n226 = Compound Arithmetic op=OR(w323, w301, w310, w299) -> (w306:bool)
            n227 = case shown="True" w306 {
              frame False {
              }
              frame True {
                n228 = shared-variable ".\\Notifiers.lvlib\\Drive Command Notifier"() -> (w332:refnum<notifier>)  [unwired: 1 in, 1 out]
                n229 = shared-variable ".\\DriverController.lvlib\\LeftStickY"(0.0 ("LeftStickY")) -> ()  [unwired: 1 in, 1 out]
                n230 = shared-variable ".\\Notifiers.lvlib\\Gear Command Notifier"() -> (w335:refnum<notifier>)  [unwired: 1 in, 1 out]
                n231 = Send Notification(notification=Gear_Command."Score", notifier=w335) -> ()  [unwired: 1 in, 2 out]
                n232 = Send Notification(notification=Drive_Commands."Tank Drive", notifier=w332) -> ()  [unwired: 1 in, 2 out]
              }
            }
            n233 = Select(t=w304, s=w306, f=w305) -> (s? t:f=w303:dbl)
            n234 = Select(t=AutoStates."Leave Peg", s=w306, f=w322) -> (s? t:f=w300:T6)
            n235 = Bundle By Name(cluster=w308, "Left Encoder Init"=w303) -> (w307:T4)
            n236 = shared-variable ".\\Notifiers.lvlib\\Right"(0.0 ("LeftStickY")) -> ()  [unwired: 1 in, 1 out]
            n237 = shared-variable ".\\Notifiers.lvlib\\Left"(0.0 ("LeftStickY")) -> ()  [unwired: 1 in, 1 out]
          }
        }
      }
      frame "Hopper Shoot" {
        n238 = shared-variable ".\\Auto Variables.lvlib\\Blue Alliance?"() -> (w340:bool)  [unwired: 1 in, 1 out]
        n239 = Unbundle By Name(w336) -> ("Gear"=w338:bool)
        n240 = Not(x=w345) -> (.not. x?=w343:bool)
        n241 = Not(x=w338) -> (.not. x?=w351:bool)
        n242 = Not(x=w340) -> (.not. x?=w339:bool)
        n243 = Or(x=w339, y=w338) -> (x .or. y?=w337:bool)
        n244 = call <userlib>:"Pulse_Stretch_&_Delay.vi"("Delay (sec)"=2.3, "In"=w343, "Width (sec)"=0.1) -> ("Out"=w341:bool)  [unwired: 2 in]
        n245 = disable-structure shown="Enabled" {
          disable-tunnel: w341 -> [w365 _]
          disable-tunnel: w337 -> [w355 _]
          frame Disabled {
            n246 = shared-variable ".\\Sensors.lvlib\\Right Encoder Distance"() -> (w362:dbl)  [unwired: 1 in, 1 out]
            n247 = shared-variable ".\\Vision Variables.lvlib\\Boiler Target Lock"() -> (w366:bool)  [unwired: 1 in, 1 out]
            n248 = shared-variable ".\\Notifiers.lvlib\\Left"(0.0 ("Turning Distance")) -> ()  [unwired: 1 in, 1 out]
            n249 = feedback #5(w362) -> (w375:dbl)
            n250 = Select(t=w362, s=w365, f=w375) -> (s? t:f=w374:dbl)
            n251 = feedback-in #5(w374) -> ()
            n252 = shared-variable ".\\Vision Variables.lvlib\\Boiler Found"() -> (w364:bool)  [unwired: 1 in, 1 out]
            n253 = Subtract(x=w374, y=1.5) -> (x-y=w372:dbl)
            n254 = Less?(x=w362, y=w372) -> (x < y?=w357:bool)
            n255 = Or(x=w355, y=w357) -> (x .or. y?=w356:bool)
            n256 = And(x=w366, y=w356) -> (x .and. y?=w360:bool)
            n257 = And(x=w364, y=w356) -> (x .and. y?=w363:bool)
            n258 = call <userlib>:"Stable.vi"("Eval Period (sec)"=0.25, "Signal Input"=w360) -> ("Stable"=w358:bool)  [unwired: 9 in]
            n259 = call <userlib>:"Stable.vi"("Eval Period (sec)"=2.5 ("Fall Delay(sec)"), "Signal Input"=w363) -> ("Stable"=w361:bool)  [unwired: 9 in]
            n260 = shared-variable ".\\Vision Variables.lvlib\\TargetTracking"(w356) -> ()  [unwired: 1 in, 1 out]
            n261 = Or(x=w361, y=w358) -> (x .or. y?=w376:bool)
            n262 = Select(t=0.0, s=w356, f=-0.75) -> (s? t:f=w371:dbl)
            n263 = shared-variable ".\\ControlMode.lvlib\\ShootingMode"(w376) -> ()  [unwired: 1 in, 1 out]
            n264 = shared-variable ".\\Auto Variables.lvlib\\OverrideSpinUpTime"(w361) -> ()  [unwired: 1 in, 1 out]
            n265 = shared-variable ".\\Notifiers.lvlib\\Right"(w371) -> ()  [unwired: 1 in, 1 out]
          }
          frame Enabled {
            w382 = 0.4 ("Left")
            n266 = shared-variable ".\\Vision Variables.lvlib\\TargetTracking"(TRUE ("TargetTracking")) -> ()  [unwired: 1 in, 1 out]
            n267 = shared-variable ".\\Notifiers.lvlib\\Left"(w382) -> ()  [unwired: 1 in, 1 out]
            n268 = shared-variable ".\\Notifiers.lvlib\\Right"(w382) -> ()  [unwired: 1 in, 1 out]
            n269 = shared-variable ".\\Vision Variables.lvlib\\Boiler Target Lock"() -> (w379:bool)  [unwired: 1 in, 1 out]
            n270 = shared-variable ".\\Vision Variables.lvlib\\Boiler Found"() -> (w381:bool)  [unwired: 1 in, 1 out]
            n271 = call <userlib>:"Stable.vi"("Eval Period (sec)"=1.0 ("Fall Delay(sec)"), "Signal Input"=w381) -> ("Stable"=w380:bool)  [unwired: 9 in]
            n272 = Or(x=w380, y=w379) -> (x .or. y?=w378:bool)
            n273 = shared-variable ".\\ControlMode.lvlib\\ShootingMode"(w378) -> ()  [unwired: 1 in, 1 out]
          }
        }
        n274 = Boolean To (0,1)(Boolean=w343) -> (0, 1=w344:i16)
        n275 = Boolean To (0,1)(Boolean=w341) -> (0, 1=w347:i16)
        n276 = Compound Arithmetic op=AND(w340, w351, w341) -> (w349:bool)
        n277 = Boolean To (0,1)(Boolean=w349) -> (0, 1=w348:i16)
        n278 = Bundle(w344, w347, w348) -> (→"Waveform Chart":cluster{i16, i16, i16})  [unwired: 1 in]
      }
      frame "Leave Peg" {
        n279 = case shown="True" w388 {
          frame False {
          }
          frame True {
            n280 = shared-variable ".\\Notifiers.lvlib\\Drive Command Notifier"() -> (w398:refnum<notifier>)  [unwired: 1 in, 1 out]
            n281 = shared-variable ".\\Auto_QCP.lvlib\\Backup_Distance"() -> (w396:dbl)  [unwired: 1 in, 1 out]
            n282 = shared-variable ".\\ControlMode.lvlib\\Drive Distance Dist"(w396) -> ()  [unwired: 1 in, 1 out]
            n283 = Send Notification(notification=Drive_Commands."Drive Distance", notifier=w398) -> ()  [unwired: 1 in, 2 out]
          }
        }
        n284 = shared-variable ".\\Auto_QCP.lvlib\\Raise_Gear_Manip_Time"() -> (w384:dbl)  [unwired: 1 in, 1 out]
        n285 = call <userlib>:"Pulse_Stretch_&_Delay.vi"("Delay (sec)"=w384, "In"=w388, "Width (sec)"=0.1) -> ("Out"=w385:bool)  [unwired: 2 in]
        n286 = case shown="True" w385 {
          frame False {
          }
          frame True {
            n287 = shared-variable ".\\Vision Variables.lvlib\\Boiler Target Lock"() -> (w393:bool)  [unwired: 1 in, 1 out]
            n288 = shared-variable ".\\Notifiers.lvlib\\Gear Command Notifier"() -> (w395:refnum<notifier>)  [unwired: 1 in, 1 out]
            n289 = Send Notification(notification=Gear_Command."Home", notifier=w395) -> ()  [unwired: 1 in, 2 out]
            n290 = shared-variable ".\\ControlMode.lvlib\\ShootingMode"(w393) -> ()  [unwired: 1 in, 1 out]
          }
        }
        n291 = shared-variable ".\\ControlMode.lvlib\\Turning Distance"(0.0 ("Turning Distance")) -> ()  [unwired: 1 in, 1 out]
      }
      frame "Crash Adjustment" {
        n292 = feedback #6() -> (w406:dbl)  [unwired: 1 in]
        n293 = case shown="True" w407 {
          tunnel: [w413 w415] -> w405
          tunnel: w406 -> [w413 _]
          frame False {
          }
          frame True {
            n294 = shared-variable ".\\Auto_QCP.lvlib\\Backup_Crash_Distance"() -> (w414:dbl)  [unwired: 1 in, 1 out]
            n295 = shared-variable ".\\Notifiers.lvlib\\Drive Command Notifier"() -> (w418:refnum<notifier>)  [unwired: 1 in, 1 out]
            n296 = shared-variable ".\\ControlMode.lvlib\\Drive Distance Dist"(w414) -> ()  [unwired: 1 in, 1 out]
            n297 = shared-variable ".\\Sensors.lvlib\\Left Encoder"() -> (w416:dbl)  [unwired: 1 in, 1 out]
            n298 = Send Notification(notification=Drive_Commands."Drive Distance", notifier=w418) -> ()  [unwired: 1 in, 2 out]
            n299 = Add(x=w416, y=w414) -> (x+y=w415:dbl)
          }
        }
        n300 = feedback-in #6(w405) -> ()
        n301 = shared-variable ".\\Sensors.lvlib\\Left Encoder"() -> (w403:dbl)  [unwired: 1 in, 1 out]
        n302 = Subtract(x=w403, y=w405) -> (x-y=w404:dbl)
        n303 = Absolute Value(x=w404) -> (abs(x)=w402:dbl)
        n304 = Less?(x=w402, y=10.0) -> (x < y?=w400:bool)
        n305 = Select(t=AutoStates."Gear Cam Placement", s=w400, f=w409) -> (s? t:f=w408:T6)
      }
      frame "Early Left Shot" {
        w429 = 0.0 ("LeftStickY")
        n306 = shared-variable ".\\DriverController.lvlib\\LeftStickY"(w429) -> ()  [unwired: 1 in, 1 out]
        n307 = shared-variable ".\\DriverController.lvlib\\RightStickX"(w429) -> ()  [unwired: 1 in, 1 out]
        n308 = shared-variable ".\\Vision Variables.lvlib\\Boiler Target Lock"() -> (w428:bool)  [unwired: 1 in, 1 out]
        n309 = call <userlib>:"Pulse_Stretch_&_Delay.vi"("Delay (sec)"=1.0, "In"=w425, "Width (sec)"=4.0) -> ("Out"=w426:bool)  [unwired: 2 in]
        n310 = Or(x=w428, y=w426) -> (x .or. y?=w423:bool)
        n311 = call <userlib>:"Pulse_Stretch_&_Delay.vi"("Delay (sec)"=5.5, "In"=w425, "Width (sec)"=0.1) -> ("Out"=w420:bool)  [unwired: 2 in]
        n312 = shared-variable ".\\Vision Variables.lvlib\\TargetTracking"(TRUE ("TargetTracking")) -> ()  [unwired: 1 in, 1 out]
        n313 = Not(x=w420) -> (.not. x?=w419:bool)
        n314 = And(x=w419, y=w423) -> (x .and. y?=w421:bool)
        n315 = shared-variable ".\\ControlMode.lvlib\\ShootingMode"(w421) -> ()  [unwired: 1 in, 1 out]
        n316 = Select(t=AutoStates."Gear Cam Placement", s=w420, f=w433) -> (s? t:f=w434:T6)
      }
    }
    n317 = node-c288() -> ()  [unwired: 1 in, 1 out]
  }
  n318 = node-c288(w29) -> ()  [unwired: 1 out]
